vi "Q14070-Z120主界面.vi"() -> ()   [LabVIEW 2013]
uses:
  PCI8622_32.dll
  <vilib>/printing/EasyPrintingControls.llb/report_type.ctl
  <vilib>/Utility/NIReport.llb/NI_ReportGenerationCore.lvlib
  <vilib>/printing/EasyPrintingControls.llb/contents.ctl
  <vilib>/Utility/NIReport.llb/NI_report.lvclass
  <vilib>/printing/EasyPrinting.llb/Easy Print VI Panel or Documentation (path).vi
panel:
  out "电压值":dbl format="%#_4g"
  in  "压力零点标定":dbl=1.7 format="%#_4g"
  out "右压力换向(N)":dbl=5000.0 format="%#.2f"
  out "左压力换向(N)":dbl=5000.0 format="%#.2f"
  out "右压力换向":bool
  out "左压力换向":bool
  out "气缸启用":dbl
  in  "型号数量":i32=2
  in  "光幕报警使能 2":bool
  in  "光幕报警工步":dbl
  out "光幕报警提示":string
  out "顶升压力":dbl
  out "右伺服顶升位置":dbl format="%#.2f"
  out "左伺服顶升位置":dbl format="%#.2f"
  out "右顶升压力合格":bool
  out "左顶升压力合格":bool
  out "保压时间":dbl
  out "error out":errorcluster
  out "右伺服压入深度上限(mm)":dbl format="%#.2f"
  out "右伺服压入深度下限(mm)":dbl format="%#.2f"
  out "右伺服压入力上限(N)":dbl format="%#.2f"
  out "右伺服压入力下限(N)":dbl format="%#.2f"
  out "左伺服压入深度上限(mm)":dbl format="%#.2f"
  out "左伺服压入深度下限(mm)":dbl format="%#.2f"
  out "左伺服压入力上限(N)":dbl format="%#.2f"
  out "左伺服压入力下限(N)":dbl format="%#.2f"
  out "查询上序完成":bool
  out "上序合格":bool
  out "上序完成":bool
  out "本序完成":bool
  out "本序合格":bool
  in  "产品ID字符位数":dbl
  out "压力报警1":bool
  out "压力报警2":bool
  out "伺服慢进速度":dbl
  out "右伺服慢进位置":dbl format="%#.2f"
  out "左伺服慢进位置":dbl format="%#.2f"
  out "JSSJ":string
  out "FGCS":string
  out "KSSJ":string
  out "右压力参数组":dbl[](array[numeric])
  out "右位移参数组":dbl[](array[numeric])
  out "左压力参数组":dbl[](array[numeric])
  out "左位移参数组":dbl[](array[numeric])
  out "右伺服设定走位":dbl
  out "左伺服设定走位":dbl
  out "程序选择-2":bool
  out "程序选择-1":bool
  out "工步提示2":string
  out "工步提示1":string
  in  "报警工步号":u32 caption="工步号1"
  out "报警提示":string
  in  "自动工步号":u32 caption="工步号1"
  out "自动工步提示":string
  in  "产品ID":string="201209190001"
  out "员工ID":string
  out "员工姓名":string
  in  "电动缸全回零":bool
  in  "电动缸全复位":bool
  out "右伺服快进位置":dbl format="%#.2f"
  out "左伺服快进位置":dbl format="%#.2f"
  out "伺服快进速度":dbl
  out "参数保存错误":errorcluster
  out "传感器保存错误":errorcluster
  out "左实时压力(N)":dbl format="%#.3f"
  out "左实时位移(mm)":dbl=10000.0 format="%#.2f"
  out "右实时位移(mm)":dbl=10000.0 format="%#.2f"
  out "右实时压力(N)":dbl format="%#.3f"
  out "区域最小压力(N)":dbl format="%#.3f"
  out "监控点最大压力(N)":dbl format="%#.3f"
  out "监控点最小压力(N)":dbl format="%#.3f"
  out "区域最大压力(N)":dbl format="%#.3f"
  out "区域最小位移(mm)":dbl format="%#.1f"
  out "区域最大位移(mm)":dbl format="%#.1f"
  in  "左工步号2900":u32 caption="工步号1"
  in  "右工步号2700":u32 caption="工步号"
  in  "报警清除":bool
  in  "参数加载":bool
  in  "型号选择":u32(ring) items=["J706", "J709", "J728"]
  out "参数加载错误":errorcluster
  in  "停止":bool
  out "ADODB._Connection Out":refnum<k7>
  out "参数查询错误":errorcluster
  in  "联线按钮":bool
  out "通讯状态":bool
  in  "选项卡控件":T1(tab)
  out "右区域最大压力(N)":dbl
  out "右区域最小压力(N)":dbl
  out "左区域最大压力(N)":dbl
  out "左区域最小压力(N)":dbl
  out "右实测压入压力(N)":dbl format="%#.1f"
  out "左实测压入压力(N)":dbl format="%#.1f"
  out "左压力位移曲线":cluster{"Y":dbl[], "Y":dbl[]}[](graph)=[{"Y"=array[1892 elements], "Y"=array[1892 elements]}, {"Y"=[120.0, 145.0, 145.0, 120.0, 120.0], "Y"=[0.0, 0.0, 4000.0, 4000.0, 0.0]}] caption="XY图"
  out "右压力位移曲线":cluster{"Y":dbl[], "Y":dbl[]}[](graph)=[{"Y"=array[1892 elements], "Y"=array[1892 elements]}, {"Y"=[120.0, 145.0, 145.0, 120.0, 120.0], "Y"=[0.0, 0.0, 4000.0, 4000.0, 0.0]}] caption="XY图"
  out "左实测监控点压力(N)":dbl format="%#.3f"
  out "左实测压入位移(mm)":dbl format="%#.1f"
  out "右实测压入位移(mm)":dbl format="%#.1f"
  out "右实测监控点压力(N)":dbl format="%#.3f"
  out "监控点位移(mm)":dbl format="%#.2f"
  out "左压装合格":bool
  out "左压装不合格":bool
  out "右压装不合格":bool
  out "右压装合格":bool
  out "右电动缸零位":bool
  out "左电动缸下限":bool
  out "右气缸下降":bool
  out "右气缸上升":bool
  out "右气缸下位":bool
  out "右气缸上位":bool
  out "左气缸上升":bool
  out "左气缸下降":bool
  out "左气缸上位":bool
  out "左气缸下位":bool
  out "左电动缸零位":bool
  out "右电动缸上限":bool
  out "右电动缸下限":bool
  out "左电动缸上限":bool
  in  "顶升气缸上升-右":bool
  in  "顶升气缸下降-右":bool
  in  "顶升气缸上升-左":bool
  in  "顶升气缸下降-左":bool
  out "启动2按钮":bool
  out "启动1按钮":bool
  out "手动/自动":bool
  out "复位按钮":bool
  in  "电动缸下降-右":bool
  in  "电动缸上升-右":bool
  in  "电动缸下降-左":bool
  in  "电动缸上升-左":bool
  in  "电动缸回零-右":bool
  in  "电动缸回零-左":bool
  in  "电动缸复位-左":bool
  in  "电动缸复位-右":bool
  out "急停按钮":bool
  out "安全光幕":bool
  out "气压报警":bool
  in  "光幕报警使能":bool
  in  "右伺服设定走位":dbl caption="右伺服设定走位负值"
  in  "左伺服设定走位":dbl caption="左伺服设定走位负值"
  in  "电动缸绝对移动调试-右":bool
  in  "电动缸绝对移动调试-左":bool
  out "左伺服实时位置":dbl
  out "右伺服实时位置":dbl
  in  "电动缸复位-右 2":bool
  in  "电动缸复位-左 2":bool
  in  "电动缸回零-左 2":bool
  in  "电动缸回零-右 2":bool
  in  "电动缸下降-右 2":bool
  in  "电动缸上升-右 2":bool
  in  "电动缸下降-左 2":bool
  in  "电动缸上升-左 2":bool
  out "J709减震套批次号输入成功":bool
  out "J706右减震套批次号输入成功":bool
  out "J706左减震套批次号输入成功":bool
  in  "J709减震套批次号":string
  in  "J706右减震套批次号":string
  in  "J706左减震套批次号":string
  in  "传感器参数保存":bool
  in  "压力1零点偏移值":dbl format="%#.3f"
  in  "压力1比例偏移值":dbl format="%#.3f"
  in  "左位移比例偏移值":dbl format="%#.3f"
  in  "左位移零点偏移值":dbl format="%#.3f"
  in  "压力2零点偏移值":dbl format="%#.3f"
  in  "压力2比例偏移值":dbl format="%#.3f"
  in  "右位移比例偏移值":dbl format="%#.3f"
  in  "右位移零点偏移值":dbl format="%#.3f"
  in  "参数保存":bool
  in  "参数查询":bool
  in  "参数列表":string[][](table)
  # "压减震套"
  # "Copying (C) 2014 湖北唯思凌科装备制造有限公司 版权所有"
  # "此界面供伺服定位用，正常生产时 禁止操作！！！"
  # "批次号输入成功"
  # "传感器校验区"
  # "关于传感器校验：\n1、传感器校验需要由具备资质的单位或部门进行校验。\n2、具备权限的用户才能够修改传感器校验参数和试验参数。\n3、修改校验参数方法：先将比例偏移置为1，修改零点偏移，使零点值与校验的传感器一致；然后根据增幅调整比例偏移。"
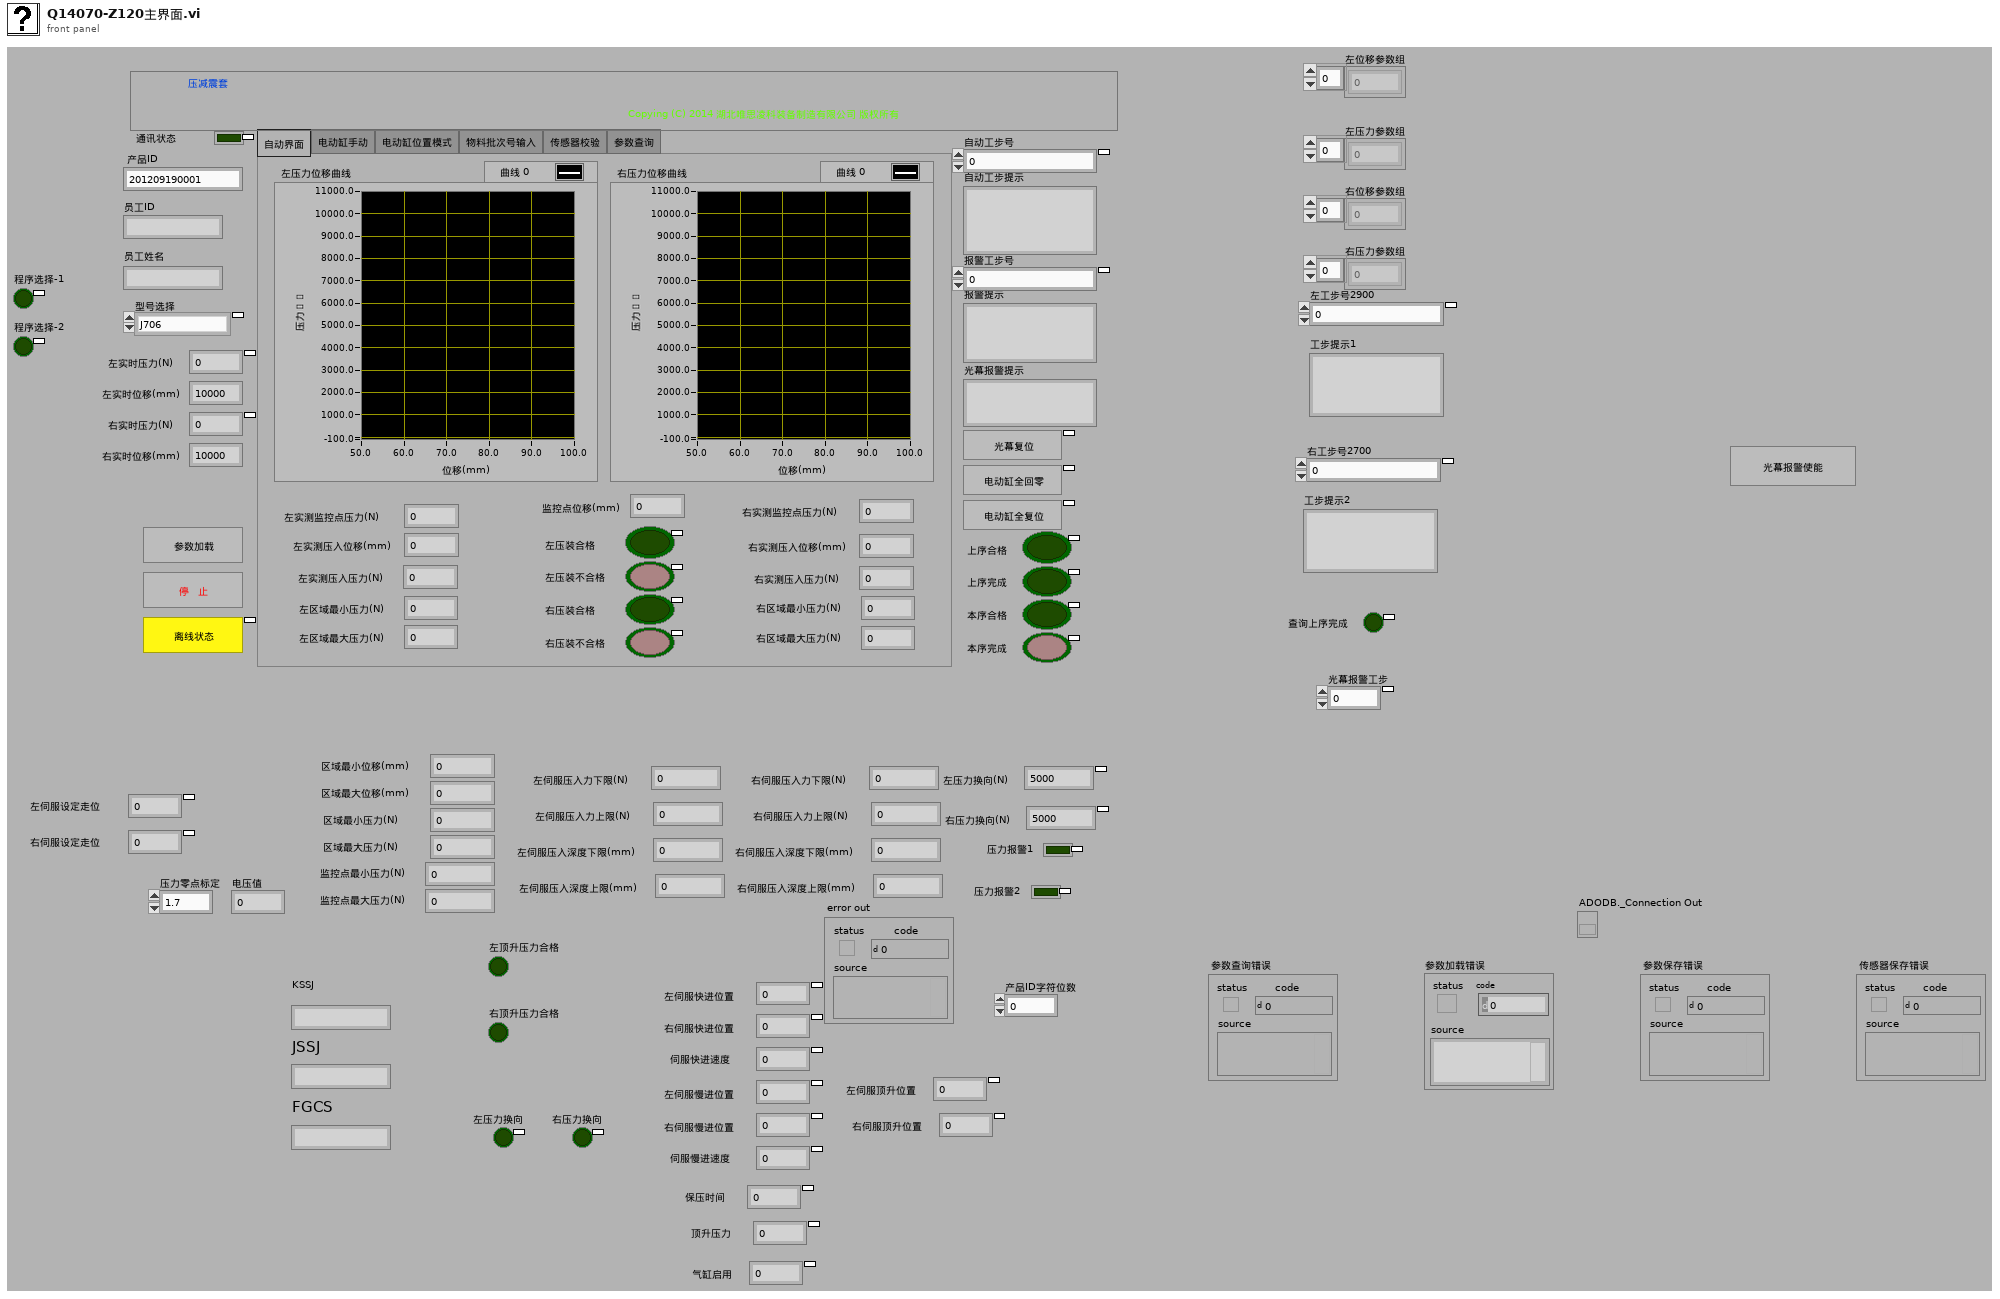
[diagram p1: front panel]
types:
  T1 = enum32{"自动界面", "电动缸手动", "电动缸位置模式", "物料批次号输入", "传感器校验", "参数查询"}
  T2 = typedef "NI_ReportGenerationCore.lvlib/report_type.ctl" = u16
  T3 = typedef "NI_ReportGenerationCore.lvlib/contents.ctl" = u16
  T4 = typedef "imagedata.ctl" = cluster{"image type":i32, "image depth":i32, "image":u8[], "mask":u8[], "colors":u32[], "Rectangle":cluster{"left":i16, "top":i16, "right":i16, "bottom":i16}}
  T5 = enum32{"invalid app kind", "Development System", "Run Time System", "Student Edition", "Embedded LabVIEW", "Evaluation", "Custom"}
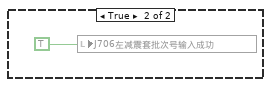
[diagram p3: hidden frame]
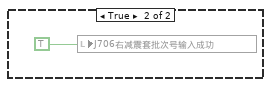
[diagram p4: hidden frame]
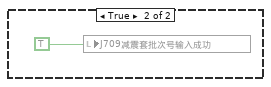
[diagram p5: hidden frame]
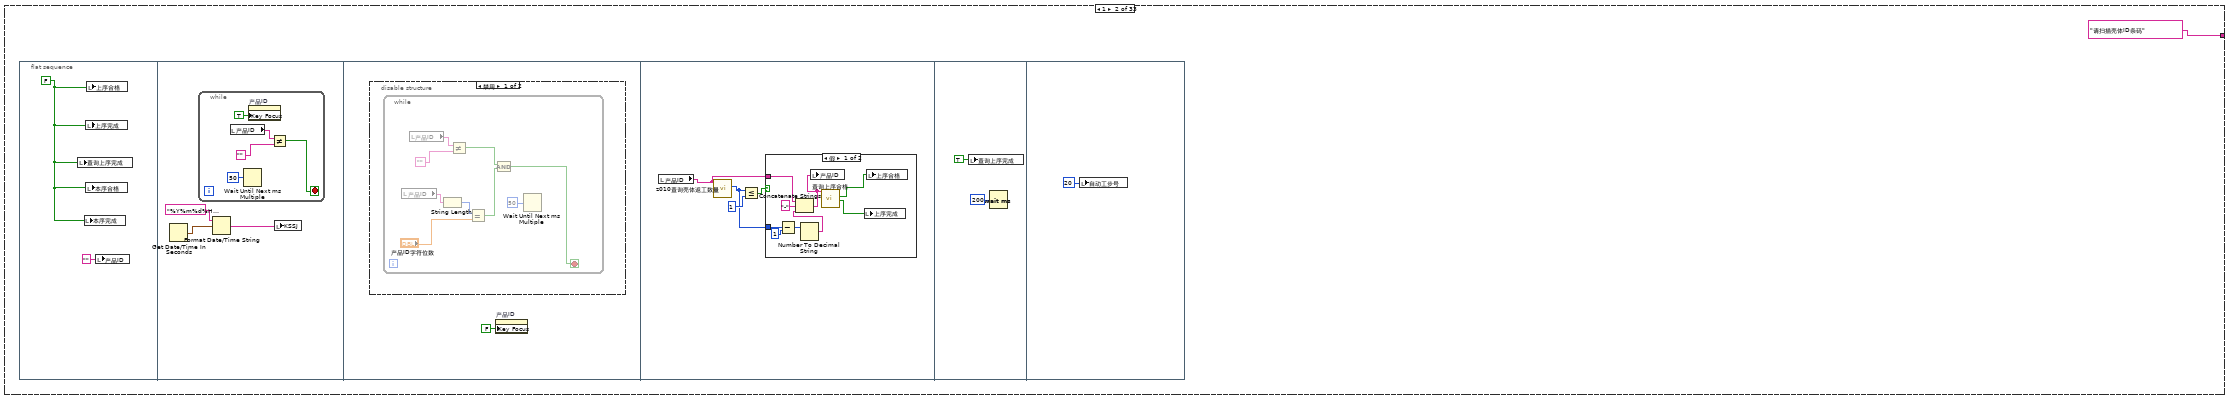
[diagram p8: hidden frame]
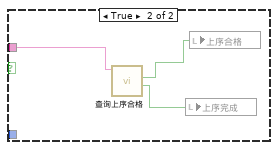
[diagram p10: hidden frame]
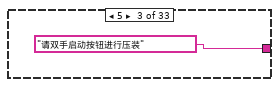
[diagram p11: hidden frame]
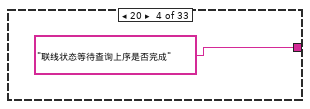
[diagram p12: hidden frame]
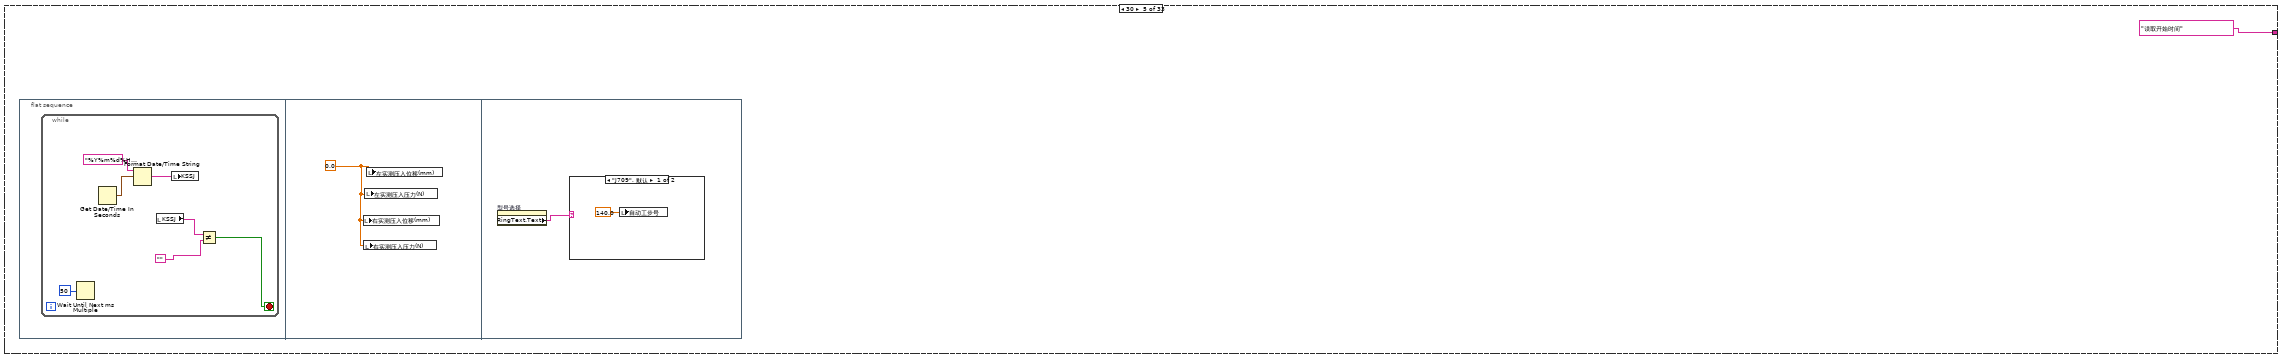
[diagram p13: hidden frame]
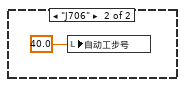
[diagram p14: hidden frame]
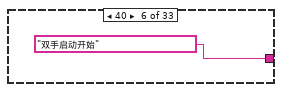
[diagram p15: hidden frame]
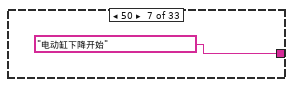
[diagram p16: hidden frame]
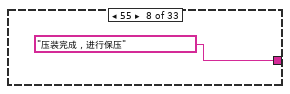
[diagram p17: hidden frame]
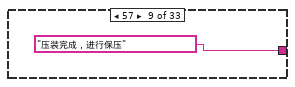
[diagram p18: hidden frame]
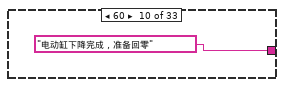
[diagram p19: hidden frame]
diagram:
  n1 = disable-structure shown="禁用" {
    frame Disabled {
      n2 = while {
        stop <- FALSE stop-if-true
        n3 = local read "右实时压力(N)"() -> (w10:dbl)
        n4 = local read "右工步号2700"() -> (w6:u32)
        n5 = local read "左实时压力(N)"() -> (w16:dbl)
        n6 = local read "左工步号2900"() -> (w18:u32)
        n7 = Greater Or Equal?(x=w16, y=1500.0) -> (x >= y?=w13:bool)
        n8 = Equal?(x=w18, y=u32 45) -> (x = y?=w14:bool)
        n9 = Greater Or Equal?(x=w10, y=1500.0) -> (x >= y?=w9:bool)
        n10 = Equal?(x=w6, y=u32 45) -> (x = y?=w5:bool)
        n11 = Compound Arithmetic op=AND(w5, w9) -> (→"右顶升压力合格":bool)
        n12 = Compound Arithmetic op=AND(w14, w13) -> (→"左顶升压力合格":bool)
      }
    }
    frame Enabled {
    }
  }
  n13 = while {
    stop <- w21 stop-if-true
    n14 = property on="型号选择" class="Ring (严格)"() -> ("RingText.Text"=w19:string)  [unwired: 2 in, 2 out]
    n15 = local read "停止"() -> (w21:bool)
    n16 = Wait Until Next ms Multiple(millisecond multiple=u32 50 ("毫秒倍数")) -> ()  [unwired: 1 out]
    n17 = case shown="\"J728\"" w19 {
      frame "J709", Default {
        n18 = local read "右工步号2700"() -> (w22:u32)
        n19 = case shown="20" w22 {
          frame 0, Default {
          }
          frame 20 {
            n20 = flat-sequence {
              tunnel: [w27] -> w23
              tunnel: [w34] -> w25
              tunnel: [w33] -> w24
              tunnel: w23 -> [w32]
              tunnel: w25 -> [w52]
              tunnel: w24 -> [w51]
              frame #0 {
                w26 = FALSE ("压装合格2")
                n21 = local write "右压装合格"(w26) -> ()
                n22 = local write "右压装不合格"(w26) -> ()
              }
              frame #1 {
                n23 = local read "区域最小位移(mm)"() -> (w31:dbl)
                n24 = local read "区域最大位移(mm)"() -> (w30:dbl)
                n25 = local read "区域最小压力(N)"() -> (w29:dbl)
                n26 = local read "区域最大压力(N)"() -> (w28:dbl)
                n27 = call "区域曲线.vi"("区域最大压力(N)"=w28, "区域最小压力(N)"=w29, "区域最大位移(mm)"=w30, "区域最小位移(mm)"=w31) -> ("区域曲线"=w27:cluster{dbl[], dbl[]})  [unwired: 7 in]
              }
              frame #2 {
                w35 = dbl[] []
                n28 = while {
                  shift-right: [w46] -> w34
                  shift-left: w35 -> [w47]
                  shift-right: [w44] -> w33
                  shift-left: w35 -> [w45]
                  tunnel: w32 -> [w37]
                  stop <- w41 stop-if-true
                  n29 = local read "左实时压力(N)"() -> (w39:dbl)
                  n30 = local read "左实时位移(mm)"() -> (w38:dbl)
                  n31 = local read "右工步号2700"() -> (w43:u32)
                  n32 = Build Array (concatenate)(w47, w38) -> (w46:dbl[])
                  n33 = Build Array (concatenate)(w45, w39) -> (w44:dbl[])
                  n34 = Equal?(x=w43, y=30.0) -> (x = y?=w41:bool)
                  n35 = Bundle(w46, w44) -> (w48:cluster{dbl[], dbl[]})  [unwired: 1 in]
                  n36 = Build Array(w48, w37) -> (w36:cluster{dbl[], dbl[]}[])
                  n37 = local write "右压力位移曲线"(w36) -> ()
                  n38 = Wait Until Next ms Multiple(millisecond multiple=u32 50 ("毫秒倍数")) -> ()  [unwired: 1 out]
                }
              }
              frame #3 {
                n39 = local read "监控点位移(mm)"() -> (w53:dbl)
                n40 = local write "右压力参数组"(w51) -> ()
                n41 = local write "右位移参数组"(w52) -> ()
                n42 = Array Max & Min "数组最大值与最小值"(array=w52) -> (max value=w50:dbl)  [unwired: 3 out]
                n43 = call "压力位移插值.vi"("压力数组"=w51, "监控点位移"=w53, "位移数组"=w52) -> ("监控点压力"=w49:dbl)  [unwired: 2 in]
                n44 = local write "右实测压入位移(mm)"(w50) -> ()
                n45 = local write "右实测监控点压力(N)"(w49) -> ()
              }
              frame #4 {
                n46 = local read "右实测压入位移(mm)"() -> (w55:dbl)
                n47 = local read "右位移参数组"() -> (w57:dbl[])
                n48 = local read "右压力参数组"() -> (w56:dbl[])
                n49 = call "压力位移插值.vi"("压力数组"=w56, "监控点位移"=w55, "位移数组"=w57) -> ("监控点压力"=w54:dbl)  [unwired: 2 in]
                n50 = local write "右实测压入压力(N)"(w54) -> ()
              }
              frame #5 {
                n51 = local read "右伺服压入力上限(N)"() -> (w63:dbl)
                n52 = local read "右伺服压入深度下限(mm)"() -> (w62:dbl)
                n53 = local read "右伺服压入力下限(N)"() -> (w65:dbl)
                n54 = local read "右实测压入压力(N)"() -> (w64:dbl)
                n55 = local read "右伺服压入深度上限(mm)"() -> (w60:dbl)
                n56 = local read "右实测压入位移(mm)"() -> (w61:dbl)
                n57 = Less Or Equal?(x=w65, y=w64) -> (x <= y?=w66:bool)
                n58 = Less Or Equal?(x=w64, y=w63) -> (x <= y?=w67:bool)
                n59 = Less Or Equal?(x=w62, y=w61) -> (x <= y?=w68:bool)
                n60 = Less Or Equal?(x=w61, y=w60) -> (x <= y?=w69:bool)
                n61 = Compound Arithmetic op=AND(w66, w67, w68, w69) -> (w59:bool)
                n62 = Not(x=w59) -> (.not. x?=w58:bool)
                n63 = local write "右压装不合格"(w58) -> ()
                n64 = local write "右压装合格"(w59) -> ()
              }
              frame #6 {
                n65 = local write "右工步号2700"(40.0 ("工步2序号")) -> ()
              }
            }
          }
        }
      }
      frame "J728" {
        n66 = local read "右工步号2700"() -> (w71:u32)
        n67 = case shown="20" w71 {
          frame 0, Default {
          }
          frame 20 {
            n68 = flat-sequence {
              tunnel: [w76] -> w72
              tunnel: [w83] -> w74
              tunnel: [w82] -> w73
              tunnel: w72 -> [w81]
              tunnel: w74 -> [w101]
              tunnel: w73 -> [w100]
              frame #0 {
                w75 = FALSE ("压装合格2")
                n69 = local write "右压装合格"(w75) -> ()
                n70 = local write "右压装不合格"(w75) -> ()
              }
              frame #1 {
                n71 = local read "区域最小位移(mm)"() -> (w80:dbl)
                n72 = local read "区域最大位移(mm)"() -> (w79:dbl)
                n73 = local read "区域最小压力(N)"() -> (w78:dbl)
                n74 = local read "区域最大压力(N)"() -> (w77:dbl)
                n75 = call "区域曲线.vi"("区域最大压力(N)"=w77, "区域最小压力(N)"=w78, "区域最大位移(mm)"=w79, "区域最小位移(mm)"=w80) -> ("区域曲线"=w76:cluster{dbl[], dbl[]})  [unwired: 7 in]
              }
              frame #2 {
                w84 = dbl[] []
                n76 = while {
                  shift-right: [w95] -> w83
                  shift-left: w84 -> [w96]
                  shift-right: [w93] -> w82
                  shift-left: w84 -> [w94]
                  tunnel: w81 -> [w90]
                  stop <- w85 stop-if-true
                  n77 = local read "右实时压力(N)"() -> (w91:dbl)
                  n78 = local read "右实时位移(mm)"() -> (w88:dbl)
                  n79 = local read "右压力换向(N)"() -> (w87:dbl)
                  n80 = local read "右实时压力(N)"() -> (w86:dbl)
                  n81 = Build Array (concatenate)(w96, w88) -> (w95:dbl[])
                  n82 = Build Array (concatenate)(w94, w91) -> (w93:dbl[])
                  n83 = Greater Or Equal?(x=w86, y=w87) -> (x >= y?=w85:bool)
                  n84 = Bundle(w95, w93) -> (w97:cluster{dbl[], dbl[]})  [unwired: 1 in]
                  n85 = local write "右压力换向"(w85) -> ()
                  n86 = Build Array(w97, w90) -> (w89:cluster{dbl[], dbl[]}[])
                  n87 = local write "右压力位移曲线"(w89) -> ()
                  n88 = Wait Until Next ms Multiple(millisecond multiple=u32 50 ("毫秒倍数")) -> ()  [unwired: 1 out]
                }
              }
              frame #3 {
                n89 = local read "区域最小位移(mm)"() -> (w105:dbl)
                n90 = local read "区域最大位移(mm)"() -> (w104:dbl)
                n91 = local read "监控点位移(mm)"() -> (w108:dbl)
                n92 = local read "区域最小压力(N)"() -> (w103:dbl)
                n93 = local read "区域最大压力(N)"() -> (w102:dbl)
                n94 = local write "右压力参数组"(w100) -> ()
                n95 = local write "右位移参数组"(w101) -> ()
                n96 = Array Max & Min "数组最大值与最小值"(array=w101) -> (max value=w107:dbl)  [unwired: 3 out]
                n97 = call "压力位移插值.vi"("压力数组"=w100, "监控点位移"=w108, "位移数组"=w101) -> ("监控点压力"=w106:dbl)  [unwired: 2 in]
                n98 = call "区域判断.vi"("压力数组"=w100, "位移数组"=w101, "区域最大压力"=w102, "区域最小压力"=w103, "区域最大位移"=w104, "区域最小位移"=w105) -> ("数值 2"=→"右区域最小压力(N)":dbl, "数值"=→"右区域最大压力(N)":dbl)  [unwired: 1 in, 1 out]
                n99 = local write "右实测压入位移(mm)"(w107) -> ()
                n100 = local write "右实测监控点压力(N)"(w106) -> ()
              }
              frame #4 {
                n101 = local read "右实测压入位移(mm)"() -> (w110:dbl)
                n102 = local read "右位移参数组"() -> (w112:dbl[])
                n103 = local read "右压力参数组"() -> (w111:dbl[])
                n104 = call "压力位移插值.vi"("压力数组"=w111, "监控点位移"=w110, "位移数组"=w112) -> ("监控点压力"=w109:dbl)  [unwired: 2 in]
                n105 = local write "右实测压入压力(N)"(w109) -> ()
              }
              frame #5 {
                n106 = local read "右伺服压入力上限(N)"() -> (w118:dbl)
                n107 = local read "右伺服压入深度下限(mm)"() -> (w117:dbl)
                n108 = local read "右伺服压入力下限(N)"() -> (w120:dbl)
                n109 = local read "右实测压入压力(N)"() -> (w119:dbl)
                n110 = local read "右伺服压入深度上限(mm)"() -> (w115:dbl)
                n111 = local read "右实测压入位移(mm)"() -> (w116:dbl)
                n112 = Less Or Equal?(x=w120, y=w119) -> (x <= y?=w121:bool)
                n113 = Less Or Equal?(x=w119, y=w118) -> (x <= y?=w122:bool)
                n114 = Less Or Equal?(x=w117, y=w116) -> (x <= y?=w123:bool)
                n115 = Less Or Equal?(x=w116, y=w115) -> (x <= y?=w124:bool)
                n116 = Compound Arithmetic op=AND(w121, w122, w123, w124) -> (w114:bool)
                n117 = Not(x=w114) -> (.not. x?=w113:bool)
                n118 = local write "右压装不合格"(w113) -> ()
                n119 = local write "右压装合格"(w114) -> ()
              }
              frame #6 {
                n120 = local write "右工步号2700"(40.0 ("工步2序号")) -> ()
              }
            }
          }
        }
      }
      frame "J706" {
        n121 = local read "右工步号2700"() -> (w126:u32)
        n122 = case shown="20" w126 {
          frame 0, Default {
          }
          frame 20 {
            n123 = flat-sequence {
              tunnel: [w131] -> w127
              tunnel: [w138] -> w129
              tunnel: [w137] -> w128
              tunnel: w127 -> [w136]
              tunnel: w129 -> [w156]
              tunnel: w128 -> [w155]
              frame #0 {
                w130 = FALSE ("压装合格2")
                n124 = local write "右压装合格"(w130) -> ()
                n125 = local write "右压装不合格"(w130) -> ()
              }
              frame #1 {
                n126 = local read "区域最小位移(mm)"() -> (w135:dbl)
                n127 = local read "区域最大位移(mm)"() -> (w134:dbl)
                n128 = local read "区域最小压力(N)"() -> (w133:dbl)
                n129 = local read "区域最大压力(N)"() -> (w132:dbl)
                n130 = call "区域曲线.vi"("区域最大压力(N)"=w132, "区域最小压力(N)"=w133, "区域最大位移(mm)"=w134, "区域最小位移(mm)"=w135) -> ("区域曲线"=w131:cluster{dbl[], dbl[]})  [unwired: 7 in]
              }
              frame #2 {
                w139 = dbl[] []
                n131 = while {
                  shift-right: [w150] -> w138
                  shift-left: w139 -> [w151]
                  shift-right: [w148] -> w137
                  shift-left: w139 -> [w149]
                  tunnel: w136 -> [w145]
                  stop <- w142 stop-if-true
                  n132 = local read "右工步号2700"() -> (w141:u32)
                  n133 = local read "右实时压力(N)"() -> (w146:dbl)
                  n134 = local read "右实时位移(mm)"() -> (w143:dbl)
                  n135 = Build Array (concatenate)(w151, w143) -> (w150:dbl[])
                  n136 = Build Array (concatenate)(w149, w146) -> (w148:dbl[])
                  n137 = Equal?(x=w141, y=30) -> (x = y?=w142:bool)
                  n138 = Bundle(w150, w148) -> (w152:cluster{dbl[], dbl[]})  [unwired: 1 in]
                  n139 = Build Array(w152, w145) -> (w144:cluster{dbl[], dbl[]}[])
                  n140 = local write "右压力位移曲线"(w144) -> ()
                  n141 = Wait Until Next ms Multiple(millisecond multiple=u32 50 ("毫秒倍数")) -> ()  [unwired: 1 out]
                }
              }
              frame #3 {
                n142 = local read "区域最小位移(mm)"() -> (w160:dbl)
                n143 = local read "区域最大位移(mm)"() -> (w159:dbl)
                n144 = local read "监控点位移(mm)"() -> (w163:dbl)
                n145 = local read "区域最小压力(N)"() -> (w158:dbl)
                n146 = local read "区域最大压力(N)"() -> (w157:dbl)
                n147 = local write "右压力参数组"(w155) -> ()
                n148 = local write "右位移参数组"(w156) -> ()
                n149 = Array Max & Min "数组最大值与最小值"(array=w156) -> (max value=w162:dbl)  [unwired: 3 out]
                n150 = call "压力位移插值.vi"("压力数组"=w155, "监控点位移"=w163, "位移数组"=w156) -> ("监控点压力"=w161:dbl)  [unwired: 2 in]
                n151 = call "区域判断.vi"("压力数组"=w155, "位移数组"=w156, "区域最大压力"=w157, "区域最小压力"=w158, "区域最大位移"=w159, "区域最小位移"=w160) -> ("数值 2"=w153:dbl, "数值"=w154:dbl)  [unwired: 1 in, 1 out]
                n152 = local write "右实测压入位移(mm)"(w162) -> ()
                n153 = local write "右实测监控点压力(N)"(w161) -> ()
                n154 = local write "右区域最大压力(N)"(w154) -> ()
                n155 = local write "右区域最小压力(N)"(w153) -> ()
              }
              frame #4 {
                n156 = local read "右实测压入位移(mm)"() -> (w165:dbl)
                n157 = local read "右位移参数组"() -> (w167:dbl[])
                n158 = local read "右压力参数组"() -> (w166:dbl[])
                n159 = call "压力位移插值.vi"("压力数组"=w166, "监控点位移"=w165, "位移数组"=w167) -> ("监控点压力"=w164:dbl)  [unwired: 2 in]
                n160 = local write "右实测压入压力(N)"(w164) -> ()
              }
              frame #5 {
                n161 = local read "右伺服压入力上限(N)"() -> (w173:dbl)
                n162 = local read "右伺服压入深度下限(mm)"() -> (w172:dbl)
                n163 = local read "右伺服压入力下限(N)"() -> (w175:dbl)
                n164 = local read "右实测压入压力(N)"() -> (w174:dbl)
                n165 = local read "右伺服压入深度上限(mm)"() -> (w170:dbl)
                n166 = local read "右实测压入位移(mm)"() -> (w171:dbl)
                n167 = Less Or Equal?(x=w175, y=w174) -> (x <= y?=w176:bool)
                n168 = Less Or Equal?(x=w174, y=w173) -> (x <= y?=w177:bool)
                n169 = Less Or Equal?(x=w172, y=w171) -> (x <= y?=w178:bool)
                n170 = Less Or Equal?(x=w171, y=w170) -> (x <= y?=w179:bool)
                n171 = Compound Arithmetic op=AND(w176, w177, w178, w179) -> (w169:bool)
                n172 = Not(x=w169) -> (.not. x?=w168:bool)
                n173 = local write "右压装不合格"(w168) -> ()
                n174 = local write "右压装合格"(w169) -> ()
              }
              frame #6 {
                n175 = local write "右工步号2700"(40.0 ("工步2序号")) -> ()
              }
            }
          }
        }
      }
    }
  }
  n176 = while {
    stop <- w183 stop-if-true
    n177 = property on="型号选择" class="Ring (严格)"() -> ("RingText.Text"=w181:string)  [unwired: 2 in, 2 out]
    n178 = Wait Until Next ms Multiple(millisecond multiple=u32 50 ("毫秒倍数")) -> ()  [unwired: 1 out]
    n179 = local read "停止"() -> (w183:bool)
    n180 = case shown="\"J706\"" w181 {
      frame "J709", Default {
        n181 = local read "左工步号2900"() -> (w184:u32)
        n182 = case shown="20" w184 {
          frame 0, Default {
          }
          frame 20 {
            n183 = flat-sequence {
              tunnel: [w193] -> w187
              tunnel: [w196] -> w186
              tunnel: [w195] -> w185
              tunnel: w187 -> [w194]
              tunnel: w186 -> [w214]
              tunnel: w185 -> [w213]
              frame #0 {
                w188 = FALSE ("压装合格1")
                n184 = local write "左压装不合格"(w188) -> ()
                n185 = local write "左压装合格"(w188) -> ()
              }
              frame #1 {
                n186 = local read "区域最小位移(mm)"() -> (w192:dbl)
                n187 = local read "区域最大位移(mm)"() -> (w191:dbl)
                n188 = local read "区域最小压力(N)"() -> (w190:dbl)
                n189 = local read "区域最大压力(N)"() -> (w189:dbl)
                n190 = call "区域曲线.vi"("区域最大压力(N)"=w189, "区域最小压力(N)"=w190, "区域最大位移(mm)"=w191, "区域最小位移(mm)"=w192) -> ("区域曲线"=w193:cluster{dbl[], dbl[]})  [unwired: 7 in]
              }
              frame #2 {
                w197 = dbl[] []
                n191 = while {
                  shift-right: [w208] -> w196
                  shift-left: w197 -> [w209]
                  shift-right: [w206] -> w195
                  shift-left: w197 -> [w207]
                  tunnel: w194 -> [w199]
                  stop <- w201 stop-if-true
                  n192 = local read "左实时位移(mm)"() -> (w205:dbl)
                  n193 = local read "左工步号2900"() -> (w203:u32)
                  n194 = local read "左实时压力(N)"() -> (w204:dbl)
                  n195 = Build Array (concatenate)(w209, w205) -> (w208:dbl[])
                  n196 = Build Array (concatenate)(w207, w204) -> (w206:dbl[])
                  n197 = Equal?(x=w203, y=30.0) -> (x = y?=w201:bool)
                  n198 = Bundle(w208, w206) -> (w210:cluster{dbl[], dbl[]})  [unwired: 1 in]
                  n199 = Build Array(w210, w199) -> (w198:cluster{dbl[], dbl[]}[])
                  n200 = local write "左压力位移曲线"(w198) -> ()
                  n201 = Wait Until Next ms Multiple(millisecond multiple=u32 50 ("毫秒倍数")) -> ()  [unwired: 1 out]
                }
              }
              frame #3 {
                n202 = local read "监控点位移(mm)"() -> (w216:dbl)
                n203 = local write "左位移参数组"(w214) -> ()
                n204 = local write "左压力参数组"(w213) -> ()
                n205 = Array Max & Min "数组最大值与最小值"(array=w214) -> (max value=w212:dbl)  [unwired: 3 out]
                n206 = call "压力位移插值.vi"("压力数组"=w213, "监控点位移"=w216, "位移数组"=w214) -> ("监控点压力"=w211:dbl)  [unwired: 2 in]
                n207 = local write "左实测监控点压力(N)"(w211) -> ()
                n208 = local write "左实测压入位移(mm)"(w212) -> ()
                n209 = Wait (ms)(milliseconds to wait=u32 200 ("等待时间（毫秒）")) -> ()  [unwired: 1 out]
              }
              frame #4 {
                n210 = local read "左实测压入位移(mm)"() -> (w218:dbl)
                n211 = local read "左位移参数组"() -> (w220:dbl[])
                n212 = local read "左压力参数组"() -> (w219:dbl[])
                n213 = call "压力位移插值.vi"("压力数组"=w219, "监控点位移"=w218, "位移数组"=w220) -> ("监控点压力"=w217:dbl)  [unwired: 2 in]
                n214 = local write "左实测压入压力(N)"(w217) -> ()
              }
              frame #5 {
                n215 = local read "左实测压入压力(N)"() -> (w224:dbl)
                n216 = local read "左伺服压入力下限(N)"() -> (w232:dbl)
                n217 = local read "左伺服压入力上限(N)"() -> (w231:dbl)
                n218 = local read "左伺服压入深度下限(mm)"() -> (w225:dbl)
                n219 = local read "左实测压入位移(mm)"() -> (w221:dbl)
                n220 = local read "左伺服压入深度上限(mm)"() -> (w230:dbl)
                n221 = Less Or Equal?(x=w232, y=w224) -> (x <= y?=w229:bool)
                n222 = Less Or Equal?(x=w224, y=w231) -> (x <= y?=w228:bool)
                n223 = Less Or Equal?(x=w225, y=w221) -> (x <= y?=w227:bool)
                n224 = Less Or Equal?(x=w221, y=w230) -> (x <= y?=w226:bool)
                n225 = Compound Arithmetic op=AND(w229, w228, w227, w226) -> (w223:bool)
                n226 = Not(x=w223) -> (.not. x?=w222:bool)
                n227 = local write "左压装合格"(w223) -> ()
                n228 = local write "左压装不合格"(w222) -> ()
              }
              frame #6 {
                n229 = local write "左工步号2900"(40.0 ("工步2序号")) -> ()
              }
            }
          }
        }
      }
      frame "J728" {
        n230 = local read "左工步号2900"() -> (w234:u32)
        n231 = case shown="20" w234 {
          frame 0, Default {
          }
          frame 20 {
            n232 = flat-sequence {
              tunnel: [w243] -> w235
              tunnel: [w246] -> w237
              tunnel: [w245] -> w236
              tunnel: w235 -> [w244]
              tunnel: w237 -> [w264]
              tunnel: w236 -> [w263]
              frame #0 {
                w238 = FALSE ("压装合格1")
                n233 = local write "左压装不合格"(w238) -> ()
                n234 = local write "左压装合格"(w238) -> ()
              }
              frame #1 {
                n235 = local read "区域最小位移(mm)"() -> (w242:dbl)
                n236 = local read "区域最大位移(mm)"() -> (w241:dbl)
                n237 = local read "区域最小压力(N)"() -> (w240:dbl)
                n238 = local read "区域最大压力(N)"() -> (w239:dbl)
                n239 = call "区域曲线.vi"("区域最大压力(N)"=w239, "区域最小压力(N)"=w240, "区域最大位移(mm)"=w241, "区域最小位移(mm)"=w242) -> ("区域曲线"=w243:cluster{dbl[], dbl[]})  [unwired: 7 in]
              }
              frame #2 {
                w247 = dbl[] []
                n240 = while {
                  shift-right: [w258] -> w246
                  shift-left: w247 -> [w259]
                  shift-right: [w256] -> w245
                  shift-left: w247 -> [w257]
                  tunnel: w244 -> [w252]
                  stop <- w248 stop-if-true
                  n241 = local read "左实时位移(mm)"() -> (w255:dbl)
                  n242 = local read "左实时压力(N)"() -> (w249:dbl)
                  n243 = local read "左实时压力(N)"() -> (w254:dbl)
                  n244 = local read "左压力换向(N)"() -> (w250:dbl)
                  n245 = Build Array (concatenate)(w259, w255) -> (w258:dbl[])
                  n246 = Build Array (concatenate)(w257, w254) -> (w256:dbl[])
                  n247 = Greater Or Equal?(x=w249, y=w250) -> (x >= y?=w248:bool)
                  n248 = local write "左压力换向"(w248) -> ()
                  n249 = Bundle(w258, w256) -> (w260:cluster{dbl[], dbl[]})  [unwired: 1 in]
                  n250 = Build Array(w260, w252) -> (w251:cluster{dbl[], dbl[]}[])
                  n251 = local write "左压力位移曲线"(w251) -> ()
                  n252 = Wait Until Next ms Multiple(millisecond multiple=u32 50 ("毫秒倍数")) -> ()  [unwired: 1 out]
                }
              }
              frame #3 {
                n253 = local read "监控点位移(mm)"() -> (w272:dbl)
                n254 = local read "区域最小压力(N)"() -> (w266:dbl)
                n255 = local read "区域最大压力(N)"() -> (w265:dbl)
                n256 = local read "区域最小位移(mm)"() -> (w268:dbl)
                n257 = local read "区域最大位移(mm)"() -> (w267:dbl)
                n258 = local write "左位移参数组"(w264) -> ()
                n259 = local write "左压力参数组"(w263) -> ()
                n260 = Array Max & Min "数组最大值与最小值"(array=w264) -> (max value=w270:dbl)  [unwired: 3 out]
                n261 = call "压力位移插值.vi"("压力数组"=w263, "监控点位移"=w272, "位移数组"=w264) -> ("监控点压力"=w269:dbl)  [unwired: 2 in]
                n262 = call "区域判断.vi"("压力数组"=w263, "位移数组"=w264, "区域最大压力"=w265, "区域最小压力"=w266, "区域最大位移"=w267, "区域最小位移"=w268) -> ("数值 2"=→"左区域最小压力(N)":dbl, "数值"=→"左区域最大压力(N)":dbl)  [unwired: 1 in, 1 out]
                n263 = local write "左实测监控点压力(N)"(w269) -> ()
                n264 = local write "左实测压入位移(mm)"(w270) -> ()
                n265 = Wait (ms)(milliseconds to wait=u32 200 ("等待时间（毫秒）")) -> ()  [unwired: 1 out]
              }
              frame #4 {
                n266 = local read "左实测压入位移(mm)"() -> (w274:dbl)
                n267 = local read "左位移参数组"() -> (w276:dbl[])
                n268 = local read "左压力参数组"() -> (w275:dbl[])
                n269 = call "压力位移插值.vi"("压力数组"=w275, "监控点位移"=w274, "位移数组"=w276) -> ("监控点压力"=w273:dbl)  [unwired: 2 in]
                n270 = local write "左实测压入压力(N)"(w273) -> ()
              }
              frame #5 {
                n271 = local read "左实测压入压力(N)"() -> (w280:dbl)
                n272 = local read "左伺服压入力下限(N)"() -> (w288:dbl)
                n273 = local read "左伺服压入力上限(N)"() -> (w287:dbl)
                n274 = local read "左伺服压入深度下限(mm)"() -> (w281:dbl)
                n275 = local read "左实测压入位移(mm)"() -> (w277:dbl)
                n276 = local read "左伺服压入深度上限(mm)"() -> (w286:dbl)
                n277 = Less Or Equal?(x=w288, y=w280) -> (x <= y?=w285:bool)
                n278 = Less Or Equal?(x=w280, y=w287) -> (x <= y?=w284:bool)
                n279 = Less Or Equal?(x=w281, y=w277) -> (x <= y?=w283:bool)
                n280 = Less Or Equal?(x=w277, y=w286) -> (x <= y?=w282:bool)
                n281 = Compound Arithmetic op=AND(w285, w284, w283, w282) -> (w279:bool)
                n282 = Not(x=w279) -> (.not. x?=w278:bool)
                n283 = local write "左压装合格"(w279) -> ()
                n284 = local write "左压装不合格"(w278) -> ()
              }
              frame #6 {
                n285 = local write "左工步号2900"(40.0 ("工步2序号")) -> ()
              }
            }
          }
        }
      }
      frame "J706" {
        n286 = local read "左工步号2900"() -> (w290:u32)
        n287 = case shown="20" w290 {
          frame 0, Default {
          }
          frame 20 {
            n288 = flat-sequence {
              tunnel: [w299] -> w291
              tunnel: [w302] -> w293
              tunnel: [w301] -> w292
              tunnel: w291 -> [w300]
              tunnel: w293 -> [w320]
              tunnel: w292 -> [w319]
              frame #0 {
                w294 = FALSE ("压装合格1")
                n289 = local write "左压装不合格"(w294) -> ()
                n290 = local write "左压装合格"(w294) -> ()
              }
              frame #1 {
                n291 = local read "区域最小位移(mm)"() -> (w298:dbl)
                n292 = local read "区域最大位移(mm)"() -> (w297:dbl)
                n293 = local read "区域最小压力(N)"() -> (w296:dbl)
                n294 = local read "区域最大压力(N)"() -> (w295:dbl)
                n295 = call "区域曲线.vi"("区域最大压力(N)"=w295, "区域最小压力(N)"=w296, "区域最大位移(mm)"=w297, "区域最小位移(mm)"=w298) -> ("区域曲线"=w299:cluster{dbl[], dbl[]})  [unwired: 7 in]
              }
              frame #2 {
                w303 = dbl[] []
                n296 = while {
                  shift-right: [w314] -> w302
                  shift-left: w303 -> [w315]
                  shift-right: [w312] -> w301
                  shift-left: w303 -> [w313]
                  tunnel: w300 -> [w308]
                  stop <- w306 stop-if-true
                  n297 = local read "左实时位移(mm)"() -> (w311:dbl)
                  n298 = local read "左工步号2900"() -> (w304:u32)
                  n299 = local read "左实时压力(N)"() -> (w310:dbl)
                  n300 = Build Array (concatenate)(w315, w311) -> (w314:dbl[])
                  n301 = Build Array (concatenate)(w313, w310) -> (w312:dbl[])
                  n302 = Equal?(x=w304, y=30.0) -> (x = y?=w306:bool)
                  n303 = Bundle(w314, w312) -> (w316:cluster{dbl[], dbl[]})  [unwired: 1 in]
                  n304 = Build Array(w316, w308) -> (w307:cluster{dbl[], dbl[]}[])
                  n305 = local write "左压力位移曲线"(w307) -> ()
                  n306 = Wait Until Next ms Multiple(millisecond multiple=u32 50 ("毫秒倍数")) -> ()  [unwired: 1 out]
                }
              }
              frame #3 {
                n307 = local read "监控点位移(mm)"() -> (w328:dbl)
                n308 = local read "区域最小压力(N)"() -> (w322:dbl)
                n309 = local read "区域最大压力(N)"() -> (w321:dbl)
                n310 = local read "区域最小位移(mm)"() -> (w324:dbl)
                n311 = local read "区域最大位移(mm)"() -> (w323:dbl)
                n312 = local write "左位移参数组"(w320) -> ()
                n313 = local write "左压力参数组"(w319) -> ()
                n314 = Array Max & Min "数组最大值与最小值"(array=w320) -> (max value=w326:dbl)  [unwired: 3 out]
                n315 = call "压力位移插值.vi"("压力数组"=w319, "监控点位移"=w328, "位移数组"=w320) -> ("监控点压力"=w325:dbl)  [unwired: 2 in]
                n316 = call "区域判断.vi"("压力数组"=w319, "位移数组"=w320, "区域最大压力"=w321, "区域最小压力"=w322, "区域最大位移"=w323, "区域最小位移"=w324) -> ("数值 2"=w317:dbl, "数值"=w318:dbl)  [unwired: 1 in, 1 out]
                n317 = local write "左实测监控点压力(N)"(w325) -> ()
                n318 = local write "左实测压入位移(mm)"(w326) -> ()
                n319 = Wait (ms)(milliseconds to wait=u32 200 ("等待时间（毫秒）")) -> ()  [unwired: 1 out]
                n320 = local write "左区域最大压力(N)"(w318) -> ()
                n321 = local write "左区域最小压力(N)"(w317) -> ()
              }
              frame #4 {
                n322 = local read "左实测压入位移(mm)"() -> (w330:dbl)
                n323 = local read "左位移参数组"() -> (w332:dbl[])
                n324 = local read "左压力参数组"() -> (w331:dbl[])
                n325 = call "压力位移插值.vi"("压力数组"=w331, "监控点位移"=w330, "位移数组"=w332) -> ("监控点压力"=w329:dbl)  [unwired: 2 in]
                n326 = local write "左实测压入压力(N)"(w329) -> ()
              }
              frame #5 {
                n327 = local read "左实测压入压力(N)"() -> (w336:dbl)
                n328 = local read "左伺服压入力下限(N)"() -> (w344:dbl)
                n329 = local read "左伺服压入力上限(N)"() -> (w343:dbl)
                n330 = local read "左伺服压入深度下限(mm)"() -> (w337:dbl)
                n331 = local read "左实测压入位移(mm)"() -> (w333:dbl)
                n332 = local read "左伺服压入深度上限(mm)"() -> (w342:dbl)
                n333 = Less Or Equal?(x=w344, y=w336) -> (x <= y?=w341:bool)
                n334 = Less Or Equal?(x=w336, y=w343) -> (x <= y?=w340:bool)
                n335 = Less Or Equal?(x=w337, y=w333) -> (x <= y?=w339:bool)
                n336 = Less Or Equal?(x=w333, y=w342) -> (x <= y?=w338:bool)
                n337 = Compound Arithmetic op=AND(w341, w340, w339, w338) -> (w335:bool)
                n338 = Not(x=w335) -> (.not. x?=w334:bool)
                n339 = local write "左压装合格"(w335) -> ()
                n340 = local write "左压装不合格"(w334) -> ()
              }
              frame #6 {
                n341 = local write "左工步号2900"(40.0 ("工步2序号")) -> ()
              }
            }
          }
        }
      }
    }
  }
  n342 = while {
    stop <- w348 stop-if-true
    n343 = Wait Until Next ms Multiple(millisecond multiple=u32 50 ("毫秒倍数")) -> ()  [unwired: 1 out]
    n344 = local read "自动工步号"() -> (w349:u32)
    n345 = local read "停止"() -> (w348:bool)
    n346 = case shown="0, 默认" w349 {
      tunnel: ["请扫描物料批次号" "请扫描壳体ID条码" "请双手启动按钮进行压装" "联线状态等待查询上序是否完成" "读取开始时间" "双手启动开始" "电动缸下降开始" "压装完成，进行保压" "压装完成，进行保压" "电动缸下降完成，准备回零" _ "等待左右伺服缸回零中" "" "" "" "" "" _ "" "" "" "" "" "" "" _ "" "" "" "绘制保存曲线、参数" "上传数据至服务器" "循环完成，归零" "联线状态查询上序不合格，请返修"] -> w346
      frame 0, Default {
        w350 = FALSE ("右压力换向")
        n347 = disable-structure shown="禁用" {
          frame Disabled {
            n348 = flat-sequence {
              frame #0 {
                n349 = while {
                  stop <- w354 stop-if-true
                  n350 = local read "J706左减震套批次号"() -> (w353:string)
                  n351 = local read "自动工步号"() -> (w352:u32)
                  n352 = Not Equal?(x=w353, y="") -> (x != y?=w356:bool)
                  n353 = Not Equal?(x=w352, y=0.0) -> (x != y?=w355:bool)
                  n354 = Compound Arithmetic op=OR(w356, w355) -> (w354:bool)
                  n355 = Wait Until Next ms Multiple(millisecond multiple=u32 50 ("毫秒倍数")) -> ()  [unwired: 1 out]
                }
              }
              frame #1 {
                n356 = local read "J706左减震套批次号"() -> (w362:string)
                n357 = property on="型号选择" class="Ring (严格)"() -> ("RingText.Text"=w360:string)  [unwired: 2 in, 2 out]
                n358 = call "比较批次号关键字.vi"("批次号"=w362, "外购件名称"="", "产品型号"=w360) -> ("关键字正确"=w361:bool)  [unwired: 6 in, 1 out]
                n359 = case shown="假" w361 {
                  frame False {
                    n360 = local write "J706左减震套批次号输入成功"(FALSE ("防尘罩批次号输入成功")) -> ()
                    n361 = call "显示对话框信息"("Enable"=TRUE) -> ()  [unwired: 9 in, 2 out]
                    n362 = local write "J706左减震套批次号"("") -> ()
                  }
                  frame True {
                    n363 = local write "J706左减震套批次号输入成功"(TRUE ("防尘罩批次号输入成功")) -> ()
                  }
                }
              }
              frame #2 {
                n364 = while {
                  stop <- w370 stop-if-true
                  n365 = local read "J706右减震套批次号"() -> (w369:string)
                  n366 = local read "自动工步号"() -> (w368:u32)
                  n367 = Not Equal?(x=w369, y="") -> (x != y?=w372:bool)
                  n368 = Not Equal?(x=w368, y=0.0) -> (x != y?=w371:bool)
                  n369 = Compound Arithmetic op=OR(w372, w371) -> (w370:bool)
                  n370 = Wait Until Next ms Multiple(millisecond multiple=u32 50 ("毫秒倍数")) -> ()  [unwired: 1 out]
                }
              }
              frame #3 {
                n371 = local read "J706右减震套批次号"() -> (w377:string)
                n372 = property on="型号选择" class="Ring (严格)"() -> ("RingText.Text"=w379:string)  [unwired: 2 in, 2 out]
                n373 = call "比较批次号关键字.vi"("批次号"=w377, "外购件名称"="", "产品型号"=w379) -> ("关键字正确"=w378:bool)  [unwired: 6 in, 1 out]
                n374 = case shown="假" w378 {
                  frame False {
                    n375 = local write "J706右减震套批次号输入成功"(FALSE ("防尘罩批次号输入成功")) -> ()
                    n376 = call "显示对话框信息4"("Enable"=TRUE) -> ()  [unwired: 9 in, 2 out]
                    n377 = local write "J706右减震套批次号"("") -> ()
                  }
                  frame True {
                    n378 = local write "J706右减震套批次号输入成功"(TRUE ("防尘罩批次号输入成功")) -> ()
                  }
                }
              }
              frame #4 {
                n379 = while {
                  stop <- w388 stop-if-true
                  n380 = local read "J709减震套批次号"() -> (w387:string)
                  n381 = local read "自动工步号"() -> (w385:u32)
                  n382 = Not Equal?(x=w385, y=0.0) -> (x != y?=w384:bool)
                  n383 = Not Equal?(x=w387, y="") -> (x != y?=w389:bool)
                  n384 = Wait Until Next ms Multiple(millisecond multiple=u32 50 ("毫秒倍数")) -> ()  [unwired: 1 out]
                  n385 = Compound Arithmetic op=OR(w389, w384) -> (w388:bool)
                }
              }
              frame #5 {
                n386 = local read "J709减震套批次号"() -> (w393:string)
                n387 = property on="型号选择" class="Ring (严格)"() -> ("RingText.Text"=w395:string)  [unwired: 2 in, 2 out]
                n388 = call "比较批次号关键字.vi"("批次号"=w393, "外购件名称"="", "产品型号"=w395) -> ("关键字正确"=w394:bool)  [unwired: 6 in, 1 out]
                n389 = case shown="假" w394 {
                  frame False {
                    n390 = local write "J709减震套批次号输入成功"(FALSE ("防尘罩批次号输入成功")) -> ()
                    n391 = call "显示对话框信息3"("Enable"=TRUE) -> ()  [unwired: 9 in, 2 out]
                    n392 = local write "J709减震套批次号"("") -> ()
                  }
                  frame True {
                    n393 = local write "J709减震套批次号输入成功"(TRUE ("防尘罩批次号输入成功")) -> ()
                  }
                }
              }
              frame #6 {
                n394 = local read "J706左减震套批次号输入成功"() -> (w403:bool)
                n395 = local read "J706右减震套批次号输入成功"() -> (w401:bool)
                n396 = local read "J709减震套批次号输入成功"() -> (w400:bool)
                n397 = Compound Arithmetic op=AND(w403, w401, w400) -> (w402:bool)
                n398 = case shown="真" w402 {
                  frame False {
                  }
                  frame True {
                    n399 = local write "自动工步号"(1.0 ("批次号扫描工步")) -> ()
                  }
                }
              }
            }
          }
          frame Enabled {
          }
        }
        n400 = local write "右压力换向"(w350) -> ()
        n401 = local write "左压力换向"(w350) -> ()
      }
      frame 1 {
        n402 = flat-sequence {
          frame #0 {
            w407 = FALSE ("上序合格")
            n403 = local write "查询上序完成"(w407) -> ()
            n404 = local write "本序完成"(w407) -> ()
            n405 = local write "上序完成"(w407) -> ()
            n406 = local write "本序合格"(w407) -> ()
            n407 = local write "上序合格"(w407) -> ()
            n408 = local write "产品ID"("" ("产品ID")) -> ()
          }
          frame #1 {
            n409 = Get Date/Time In Seconds() -> (seconds since 1Jan1904=w410:timestamp)
            n410 = while {
              stop <- w411 stop-if-true
              n411 = local read "产品ID"() -> (w412:string)
              n412 = Wait Until Next ms Multiple(millisecond multiple=u32 50 ("毫秒倍数")) -> ()  [unwired: 1 out]
              n413 = property on="产品ID" class="Str"("Key Focus"=TRUE ("键选中")) -> ()  [unwired: 2 in, 2 out]
              n414 = Not Equal?(x=w412, y="") -> (x != y?=w411:bool)
            }
            n415 = Format Date/Time String(time format string (%c)="%Y%m%d%H%M" ("时间格式字符串(%c)"), seconds (now)=w410) -> (date/time string=w408:string)  [unwired: 1 in]
            n416 = local write "KSSJ"(w408) -> ()
          }
          frame #2 {
            n417 = disable-structure shown="禁用" {
              frame Disabled {
                n418 = while {
                  stop <- w419 stop-if-true
                  n419 = local read "产品ID"() -> (w423:string)
                  n420 = local read "产品ID"() -> (w425:string)
                  n421 = String Length(string=w423) -> (length=w422:i32)
                  n422 = Not Equal?(x=w425, y="") -> (x != y?=w420:bool)
                  n423 = Equal?(x=w422, y="产品ID字符位数") -> (x = y?=w421:bool)
                  n424 = Compound Arithmetic op=AND(w420, w421) -> (w419:bool)
                  n425 = Wait Until Next ms Multiple(millisecond multiple=u32 50 ("毫秒倍数")) -> ()  [unwired: 1 out]
                }
              }
              frame Enabled {
              }
            }
            n426 = property on="产品ID" class="Str"("Key Focus"=FALSE ("键选中")) -> ()  [unwired: 2 in, 2 out]
          }
          frame #3 {
            n427 = local read "产品ID"() -> (w427:string)
            n428 = call "z010查询壳体返工数量.vi"("转向器总成ID"=w427) -> ("Rows Fetched"=w426:i32)  [unwired: 8 in, 2 out]
            n429 = Less Or Equal?(x=w426, y=1) -> (x <= y?=w429:bool)
            n430 = case shown="假" w429 {
              tunnel: w427 -> [w432 w439]
              tunnel: w426 -> [w435 _]
              frame False {
                n431 = Subtract(x=w435, y=1) -> (x-y=w433:i32)
                n432 = Number To Decimal String(number=w433) -> (decimal integer string=w436:string)  [unwired: 1 in]
                n433 = Concatenate Strings(w432, "-" ("字符串"), w436) -> (w430:string)
                n434 = local write "产品ID"(w430) -> ()
                n435 = call "查询上序合格.vi"("产品ID"=w430) -> ("本序已做"=w438:bool, "上序合格"=w437:bool)  [unwired: 8 in, 1 out]
                n436 = local write "上序完成"(w438) -> ()
                n437 = local write "上序合格"(w437) -> ()
              }
              frame True {
                n438 = call "查询上序合格.vi"("产品ID"=w439) -> ("本序已做"=w441:bool, "上序合格"=w440:bool)  [unwired: 8 in, 1 out]
                n439 = local write "上序完成"(w441) -> ()
                n440 = local write "上序合格"(w440) -> ()
              }
            }
          }
          frame #4 {
            n441 = local write "查询上序完成"(TRUE ("查询上序完成")) -> ()
            n442 = Wait (ms)(milliseconds to wait=u32 200 ("等待时间（毫秒）")) -> ()  [unwired: 1 out]
          }
          frame #5 {
            n443 = local write "自动工步号"(u32 20 ("自动工步号")) -> ()
          }
        }
      }
      frame 5 {
      }
      frame 20 {
      }
      frame 30 {
        n444 = flat-sequence {
          frame #0 {
            n445 = while {
              stop <- w448 stop-if-true
              n446 = Wait Until Next ms Multiple(millisecond multiple=u32 50 ("毫秒倍数")) -> ()  [unwired: 1 out]
              n447 = Get Date/Time In Seconds() -> (seconds since 1Jan1904=w453:timestamp)
              n448 = Format Date/Time String(time format string (%c)="%Y%m%d%H%M" ("时间格式字符串(%c)"), seconds (now)=w453) -> (date/time string=w452:string)  [unwired: 1 in]
              n449 = local read "KSSJ"() -> (w450:string)
              n450 = local write "KSSJ"(w452) -> ()
              n451 = Not Equal?(x=w450, y="") -> (x != y?=w448:bool)
            }
          }
          frame #1 {
            w455 = 0.0 ("左实测压入位移(mm)")
            n452 = local write "右实测压入位移(mm)"(w455) -> ()
            n453 = local write "右实测压入压力(N)"(w455) -> ()
            n454 = local write "左实测压入压力(N)"(w455) -> ()
            n455 = local write "左实测压入位移(mm)"(w455) -> ()
          }
          frame #2 {
            n456 = property on="型号选择" class="Ring (严格)"() -> ("RingText.Text"=w456:string)  [unwired: 2 in, 2 out]
            n457 = case shown="\"J709\", 默认" w456 {
              frame "J709", Default {
                n458 = local write "自动工步号"(140.0 ("内球节工步号")) -> ()
              }
              frame "J706" {
                n459 = local write "自动工步号"(40.0 ("内球节工步号")) -> ()
              }
            }
          }
        }
      }
      frame 40 {
      }
      frame 50 {
      }
      frame 55 {
      }
      frame 57 {
      }
      frame 60 {
      }
      frame 65 {
      }
      frame 70 {
      }
      frame 140 {
      }
      frame 150 {
      }
      frame 155 {
      }
      frame 157 {
      }
      frame 160 {
      }
      frame 165 {
      }
      frame 170 {
      }
      frame 180 {
      }
      frame 240 {
      }
      frame 250 {
      }
      frame 255 {
      }
      frame 257 {
      }
      frame 260 {
      }
      frame 265 {
      }
      frame 270 {
      }
      frame 280 {
      }
      frame 290 {
      }
      frame 800 {
        n460 = flat-sequence {
          tunnel: [w510] -> w499
          tunnel: [w508] -> w498
          tunnel: [w502] -> w483
          tunnel: [w500] -> w480
          tunnel: w499 -> [w517]
          tunnel: w498 -> [w516]
          tunnel: [w517] -> w497
          tunnel: [w516] -> w496
          tunnel: ["F:\\报表存储\\" ("字符串")] -> w495
          tunnel: w483 -> [w514]
          tunnel: [w514] -> w482
          tunnel: [w513] -> w481
          tunnel: w480 -> [w513]
          tunnel: w497 -> [w522]
          tunnel: w496 -> [w518]
          tunnel: w495 -> [w523]
          tunnel: [w532] -> w494
          tunnel: [w530] -> w493
          tunnel: [w528] -> w492
          tunnel: [w524] -> w491
          tunnel: w482 -> [w521]
          tunnel: w481 -> [w520]
          tunnel: w494 -> [w538]
          tunnel: [w539] -> w490
          tunnel: w493 -> [w539]
          tunnel: w492 -> [w537]
          tunnel: [w536] -> w489
          tunnel: w491 -> [w535]
          tunnel: [w534] -> w488
          tunnel: [w553] -> w487
          tunnel: w490 -> [w553]
          tunnel: w489 -> [w552]
          tunnel: [w552] -> w486
          tunnel: [w551] -> w485
          tunnel: w488 -> [w551]
          tunnel: w487 -> [w560]
          tunnel: w486 -> [w559]
          tunnel: w485 -> [w556]
          frame #0 {
            n461 = local read "产品ID"() -> (w509:string)
            n462 = Format Date/Time String(time format string (%c)="%Y%m%d" ("时间格式字符串(%c)")) -> (date/time string=w501:string)  [unwired: 2 in]
            n463 = String Subset(string=w501, offset (0)=4 ("偏移量(0)"), length (rest)=2 ("长度（剩余）")) -> (substring=w502:string)
            n464 = String Subset(string=w501, offset (0)=6 ("偏移量(0)"), length (rest)=2 ("长度（剩余）")) -> (substring=w500:string)
            n465 = call <vilib>:"Trim Whitespace.vi"("string"=w509) -> ("trimmed string"=w508:string)  [unwired: 1 in]
            n466 = String Subset(string=w501, offset (0)=0 ("偏移量(0)"), length (rest)=4 ("长度（剩余）")) -> (substring=w510:string)
          }
          frame #1 {
          }
          frame #2 {
            w519 = "\\" ("字符串")
            n467 = Concatenate Strings(w523, w522, w519, w521, w519, w520, w519) -> (w525:string)
            n468 = Concatenate Strings(w523, w522, w519, w521, w519, w520, w519) -> (w533:string)
            n469 = String To Path(string=w533) -> (path=w532:path)
            n470 = Concatenate Strings(w525, w518, ".JPG" ("字符串")) -> (w531:string)
            n471 = Concatenate Strings(w525, w518, "右.txt" ("字符串")) -> (w524:string)
            n472 = Concatenate Strings(w525, w518, "左.txt" ("字符串")) -> (w528:string)
            n473 = String To Path(string=w531) -> (path=w530:path)
          }
          frame #3 {
            n474 = call <vilib>:"Check if File or Folder Exists.vi"("path"=w538) -> ("file or folder exists?"=w540:bool)  [unwired: 8 in, 2 out]
            n475 = String To Path(string=w537) -> (path=w536:path)
            n476 = String To Path(string=w535) -> (path=w534:path)
            n477 = case shown="真" w540 {
              tunnel: w538 -> [w541 w542]
              frame False {
                n478 = Create Folder(path (use dialog)=w541) -> ()  [unwired: 2 in, 3 out]
              }
              frame True {
                n479 = flat-sequence {
                  tunnel: w542 -> [w546]
                  tunnel: [w544] -> w543
                  tunnel: w543 -> [w549]
                  frame #0 {
                    n480 = Delete(path (use dialog)=w546, entire hierarchy (F)=TRUE ("整个层次结构(F)")) -> (deleted path=w544:path)  [unwired: 3 in, 2 out]
                  }
                  frame #1 {
                    n481 = call <vilib>:"Check if File or Folder Exists.vi"("path"=w549) -> ("file or folder exists?"=w548:bool, "dup path"=w547:path)  [unwired: 8 in, 1 out]
                    n482 = case shown="假" w548 {
                      tunnel: w547 -> [w550 _]
                      frame False {
                        n483 = Create Folder(path (use dialog)=w550) -> ()  [unwired: 2 in, 3 out]
                      }
                      frame True {
                      }
                    }
                  }
                }
              }
            }
          }
          frame #4 {
            n484 = Wait Until Next ms Multiple(millisecond multiple=u32 1000 ("毫秒倍数")) -> ()  [unwired: 1 out]
          }
          frame #5 {
            n485 = flat-sequence {
              tunnel: w559 -> [w563]
              tunnel: w560 -> [w564]
              tunnel: [w564] -> w558
              tunnel: [w563] -> w557
              tunnel: w556 -> [w562]
              tunnel: [w562] -> w555
              tunnel: w558 -> [w565]
              tunnel: w557 -> [w568]
              tunnel: w555 -> [w571]
              frame #0 {
                n486 = local write "选项卡控件"(T1."自动界面" ("选项卡控件")) -> ()
              }
              frame #1 {
                n487 = local read "左位移参数组"() -> (w572:dbl[])
                n488 = local read "左压力参数组"() -> (w573:dbl[])
                n489 = local read "右位移参数组"() -> (w569:dbl[])
                n490 = local read "右压力参数组"() -> (w570:dbl[])
                n491 = disable-structure shown="禁用" {
                  disable-tunnel: w565 -> [w574 _]
                  frame Disabled {
                    w577 = T2 2 items=["快速打印", "标准报表", "HTML", "双字节", "Excel"] ("report type (Quick Print)")
                    w576 = T3 1 items=["完整前面板", "前面板可见部分", "图标、说明、前面板和程序框图", "说明信息: 使用前面板", "说明信息: 作为子VI使用", "说明信息: 完整", "说明信息: 自定义"] ("contents (complete front panel)")
                    n492 = Current VI's Path() -> (path=w575:path)
                    n493 = call-poly <vilib>:"Easy Print VI Panel or Documentation.vi"("report type (Quick Print)"=w577, "contents (complete front panel)"=w576, "VI path"=w575) -> ("error out"=w579:errorcluster, "report out"=w578:refnum<class "NI_report.lvclass">)  [unwired: 1 in, 6 out]
                    n494 = call-dynamic "Save Report to File.vi"("report in"=w578, "report file path"=w574, "error in (no error)"=w579) -> ()  [unwired: 2 in, 11 out]
                  }
                  frame Enabled {
                  }
                }
                n495 = call "导出曲线数组.vi"("压力参数"=w573, "位移参数"=w572, "file path (dialog if empty)"=w568) -> ()  [unwired: 17 in]
                n496 = call "导出曲线数组.vi"("压力参数"=w570, "位移参数"=w569, "file path (dialog if empty)"=w571) -> ()  [unwired: 17 in]
                n497 = control-ref of="本VI"() -> (w567:refnum<vi>)
                n498 = invoke class="VI" method="FP.Get Image"(reference=w567) -> ("image data"=w566:T4)  [unwired: 5 in, 5 out]
                n499 = call <vilib>:"Write JPEG File.vi"("image data"=w566, "path to JPEG file"=w565) -> ()  [unwired: 8 in, 2 out]
              }
            }
          }
          frame #6 {
            n500 = local write "自动工步号"(810.0 ("工步号")) -> ()
          }
        }
      }
      frame 810 {
        n501 = flat-sequence {
          tunnel: [w609] -> w582
          tunnel: w582 -> [w617]
          frame #0 {
            n502 = while {
              stop <- w585 stop-if-true
              n503 = Get Date/Time In Seconds() -> (seconds since 1Jan1904=w590:timestamp)
              n504 = local read "JSSJ"() -> (w587:string)
              n505 = Format Date/Time String(time format string (%c)="%Y%m%d%H%M" ("时间格式字符串(%c)"), seconds (now)=w590) -> (date/time string=w588:string)  [unwired: 1 in]
              n506 = Wait Until Next ms Multiple(millisecond multiple=u32 50 ("毫秒倍数")) -> ()  [unwired: 1 out]
              n507 = Not Equal?(x=w587, y="") -> (x != y?=w585:bool)
              n508 = local write "JSSJ"(w588) -> ()
            }
            n509 = Wait (ms)(milliseconds to wait=u32 2000 ("等待时间（毫秒）")) -> ()  [unwired: 1 out]
          }
          frame #1 {
            w607 = i16 4 ("精度(6)")
            n510 = local read "右实测压入位移(mm)"() -> (w597:dbl)
            n511 = local read "右实测压入压力(N)"() -> (w596:dbl)
            n512 = local read "左实测压入压力(N)"() -> (w598:dbl)
            n513 = local read "左实测压入位移(mm)"() -> (w599:dbl)
            n514 = local read "右压装合格"() -> (w591:bool)
            n515 = local read "左压装合格"() -> (w592:bool)
            n516 = local read "J706左减震套批次号"() -> (w602:string)
            n517 = local read "J709减震套批次号"() -> (w600:string)
            n518 = local read "J706右减震套批次号"() -> (w601:string)
            n519 = local read "员工ID"() -> (w613:string)
            n520 = local read "产品ID"() -> (w614:string)
            n521 = local read "KSSJ"() -> (w612:string)
            n522 = local read "JSSJ"() -> (w608:string)
            n523 = local read "FGCS"() -> (w611:string)
            n524 = And(x=w592, y=w591) -> (x .and. y?=w593:bool)
            n525 = Boolean To (0,1)(Boolean=w593) -> (0, 1=w616:i16)
            n526 = Number To Decimal String(number=w616, width (-)=i16 1 ("宽度(-)")) -> (decimal integer string=w594:string)
            n527 = Number To Fractional String(number=w599, precision (6)=w607) -> (F-format string=w606:string)  [unwired: 2 in]
            n528 = Number To Fractional String(number=w598, precision (6)=w607) -> (F-format string=w605:string)  [unwired: 2 in]
            n529 = Number To Fractional String(number=w597, precision (6)=w607) -> (F-format string=w604:string)  [unwired: 2 in]
            n530 = Number To Fractional String(number=w596, precision (6)=w607) -> (F-format string=w603:string)  [unwired: 2 in]
            n531 = Build Array(w614, w613, "1", w594, w612, w608, w611, "Q14070-Z120", w606, w605, w604, w603, w602, w601, w600) -> (w609:string[])
          }
          frame #2 {
            n532 = Wait (ms)(milliseconds to wait=u32 500 ("等待时间（毫秒）")) -> ()  [unwired: 1 out]
            n533 = call "数据库更新.vi"("设备号"="11", "数据"=w617) -> ()  [unwired: 13 in, 1 out]
          }
          frame #3 {
            n534 = local write "自动工步号"(820.0 ("工步号")) -> ()
          }
        }
      }
      frame 820 {
      }
      frame 900 {
      }
    }
    "自动工步提示" <- w346
  }
  n535 = while {
    stop <- w623 stop-if-true
    n536 = stacked-sequence {
      frame #0 {
        n537 = First Call?() -> (First Call?: T/F=w625:bool)
        n538 = case shown="真" w625 {
          frame False {
          }
          frame True {
            n539 = call "员工管理测试程序.vi"() -> ("员工姓名"=w631:string, "员工ID"=w630:string)  [unwired: 10 in]
            n540 = local write "员工ID"(w630) -> ()
            n541 = local write "员工姓名"(w631) -> ()
          }
        }
        n542 = Negate(x="右伺服设定走位") -> (-x=→"右伺服设定走位":dbl)
        n543 = Negate(x="左伺服设定走位") -> (-x=→"左伺服设定走位":dbl)
      }
      frame #1 {
        n544 = case shown="0, 默认" "报警工步号" {
          tunnel: ["工作正常" "气压报警，请检查气压" "压装过程触碰光幕，请复位后双手启动重新压装" "左压装不合格" "右压装不合格" "左压装压力过大报警" "右压装压力过大报警" "左伺服报警，请复位伺服电机" "右伺服报警，请复位伺服电机" "左伺服达到下极限，请复位后，手动点动上升离开下极限" "左伺服达到上极限，请复位后，手动点动下降离开上极限" "右伺服达到下极限，请复位后，手动点动上升离开下极限" "右伺服达到上极限，请复位后，手动点动下降离开上极限" "联线状态查询上序不合格，请返修"] -> w639
          frame 0, Default {
          }
          frame 1 {
          }
          frame 2 {
          }
          frame 6 {
          }
          frame 7 {
          }
          frame 8 {
          }
          frame 9 {
          }
          frame 11 {
          }
          frame 12 {
          }
          frame 21 {
          }
          frame 22 {
          }
          frame 23 {
          }
          frame 24 {
          }
          frame 41 {
          }
        }
        "报警提示" <- w639
        n545 = case shown="10" "左工步号2900" {
          tunnel: ["准备压装" "左伺服压装启动" "左伺服等待回零完成" "左伺服等待回零完成，等待右伺服回零完成" "左伺服压装中" "左伺服压装结束" "左伺服曲线采集完成" "左伺服回零开始" "左伺服回零中" "左伺服回零完成" "左伺服压装工作结束"] -> w638
          frame 0, Default {
          }
          frame 10 {
          }
          frame 15 {
          }
          frame 16 {
          }
          frame 20 {
          }
          frame 30 {
          }
          frame 40 {
          }
          frame 50 {
          }
          frame 60 {
          }
          frame 70 {
          }
          frame 80 {
          }
        }
        "工步提示1" <- w638
        n546 = case shown="80" "右工步号2700" {
          tunnel: ["准备压装" "右伺服压装启动" "右伺服等待回零完成" "右伺服等待回零完成，等待左伺服回零完成" "右伺服压装中" "右伺服压装结束" "右伺服曲线采集完成" "右伺服回零开始" "右伺服回零中" "右伺服回零完成" "右伺服压装工作结束"] -> w637
          frame 0, Default {
          }
          frame 10 {
          }
          frame 15 {
          }
          frame 16 {
          }
          frame 20 {
          }
          frame 30 {
          }
          frame 40 {
          }
          frame 50 {
          }
          frame 60 {
          }
          frame 70 {
          }
          frame 80 {
          }
        }
        "工步提示2" <- w637
        n547 = case shown="5" "光幕报警工步" {
          tunnel: ["工作正常" "压装过程触碰光幕，请再次启动"] -> w632
          frame 0, Default {
          }
          frame 5 {
          }
        }
        "光幕报警提示" <- w632
        n548 = property on="型号选择" class="Ring (严格)"() -> ("RingText.Text"=w634:string)  [unwired: 2 in, 2 out]
        n549 = case shown="\"J706\", 默认" w634 {
          frame "J706", Default {
            n550 = local write "程序选择-1"(TRUE ("程序选择-1")) -> ()
            n551 = local write "程序选择-2"(FALSE ("程序选择-2")) -> ()
          }
          frame "J709" {
            n552 = local write "程序选择-1"(FALSE ("程序选择-1")) -> ()
            n553 = local write "程序选择-2"(TRUE ("程序选择-2")) -> ()
          }
        }
      }
    }
    n554 = Wait (ms)(milliseconds to wait=u32 50 ("毫秒倍数")) -> ()  [unwired: 1 out]
    n555 = local read "停止"() -> (w623:bool)
  }
  n556 = while {
    stop <- w683 stop-if-true
    n557 = event shown="[1] \"参数查询\": 值改变" {
      selector: _ -> [_ _ _ _ _]
      dyn-events: _ -> [_ _ _ _ _]
      timeout: 500 -> [_ _ _ _ _]
      tunnel: [_ _ _ _ w807] -> w683
      event Timeout {
        n558 = event-data() -> ()  [unwired: 1 in, 3 out]
      }
      event "参数查询": Value Change {
        n559 = event-data() -> ()  [unwired: 1 in, 6 out]
        n560 = flat-sequence {
          tunnel: [w694] -> w686
          tunnel: [w691] -> w685
          tunnel: w686 -> [w698]
          tunnel: w685 -> [w697]
          frame #0 {
            n561 = call "字符串转换为数组.vi"("查询内容"=",产品型号,区域最小位移(mm),区域最大位移(mm),区域最小压力(N),区域最大压力(N),位移监控点(mm),左伺服压入力下限(N),左伺服压入力上限(N),左伺服压入深度下限(mm),左伺服压入深度上限(mm),右伺服压入力下限(N),右伺服压入力上限(N),右伺服压入深度下限(mm),右伺服压入深度上限(mm),左伺服快进位置(mm),右伺服快进位置(mm),伺服快进速度(mm/s),左伺服慢进位置(mm),右伺服慢进位置(mm),左伺服顶升位置(mm),右伺服顶升位置(mm),伺服慢进速度(mm/s),保压时间(ms),顶升压力(N),气缸启用,左压力换向(N),右压力换向(N)") -> ("列首"=w687:string[])  [unwired: 10 in]
            n562 = property on="参数列表" class="Tbl (严格)"("Row Headers[]"=w687) -> ()  [unwired: 2 in, 2 out]
          }
          frame #1 {
            w690 = 0 ("禁用的索引 (列)")
            n563 = local read "ADODB._Connection Out"() -> (w695:refnum<k7>)
            n564 = call "SQL Execute.vi"("Command Text"="select * from 测试参数表 ", "ADODB._Connection In"=w695) -> ("error out"=w694:errorcluster, "Data"=w696:string[][])  [unwired: 6 in, 2 out]
            n565 = Transpose 2D Array "二维数组转置"(2D array=w696) -> (transposed array=w691:string[][])
            n566 = Index Array(array=w691, index (col)=w690) -> (element=w692:string[])  [unwired: 1 in]
            n567 = Index Array(array=w691, index (col)=w690) -> (element=w689:string[])  [unwired: 1 in]
            n568 = property on="参数列表" class="Tbl (严格)"("Column Headers[]"=w692) -> ()  [unwired: 2 in, 2 out]
            n569 = Array Size(array=w689) -> ()  [unwired: 1 out]
          }
          frame #2 {
            n570 = local write "参数列表"(w697) -> ()
            "参数查询错误" <- w698
          }
        }
      }
      event "参数保存": Value Change {
        n571 = event-data() -> ()  [unwired: 1 in, 6 out]
        n572 = while {
          i -> [w700]
          stop <- w711 stop-if-true
          n573 = local read "型号数量"() -> (w699:i32)
          n574 = local read "参数列表"() -> (w702:string[][])
          n575 = Greater Or Equal?(x=w700, y=w699) -> (x >= y?=w711:bool)
          n576 = Wait Until Next ms Multiple(millisecond multiple=u32 100 ("毫秒倍数")) -> ()  [unwired: 1 out]
          n577 = Index Array "索引数组"(array=w702, index (col)=w700) -> (element=w703:string[])  [unwired: 1 in]
          n578 = stacked-sequence {
            seq-local: [w714 _] -> [_ w768]
            tunnel: w703 -> [w745 w773]
            tunnel: [_ w767] -> w701
            frame #0 {
              n579 = Index Array(array=w745, index #2=1 ("索引"), index #3=2 ("索引"), index #4=3 ("索引"), index #5=4 ("索引"), index #6=5 ("索引"), index #7=6 ("索引"), index #8=7 ("索引"), index #9=8 ("索引"), index #10=9 ("索引"), index #11=10 ("索引"), index #12=11 ("索引"), index #13=12 ("索引"), index #14=13 ("索引"), index #15=14 ("索引"), index #16=15 ("索引"), index #17=16 ("索引"), index #18=17 ("索引"), index #19=18 ("索引"), index #20=19 ("索引"), index #21=20 ("索引"), index #22=21 ("索引"), index #23=22 ("索引"), index #24=23 ("索引")) -> (element #2=w737:string, element #3=w736:string, element #4=w735:string, element #5=w734:string, element #6=w733:string, element #7=w732:string, element #8=w731:string, element #9=w730:string, element #10=w729:string, element #11=w728:string, element #12=w727:string, element #13=w726:string, element #14=w725:string, element #15=w724:string, element #16=w723:string, element #17=w722:string, element #18=w721:string, element #19=w720:string, element #20=w719:string, element #21=w718:string, element #22=w717:string, element #23=w716:string, element #24=w715:string)  [unwired: 2 in, 2 out]
              n580 = call "创建文本3"("区域最小位移"=w737, "区域最a大位移"=w736, "区域最小压力"=w735, "区域最大压力"=w734, "位移监控点"=w733, "左伺服压入力下限"=w732, "左伺服压入力上限"=w731, "左伺服压入深度下限"=w730, "左伺服压入深度上限"=w729, "右伺服压入力下限"=w728, "右伺服压入力上限"=w727, "右伺服压入深度下限"=w726, "右伺服压入深度上限"=w725, "左伺服快进位置"=w724, "右伺服快进位置"=w723, "伺服快进速度"=w722, "左伺服慢进位置"=w721, "右伺服慢进位置"=w720, "左伺服顶升位置"=w719, "右伺服顶升位置"=w718, "伺服慢进速度"=w717, "保压时间"=w716, "顶升压力"=w715) -> ("Result"=w714:string)  [unwired: 3 in, 1 out]
            }
            frame #1 {
              n581 = Index Array(array=w773, index #1=0 ("索引"), index #2=24 ("索引"), index #3=25 ("索引"), index #4=26 ("索引")) -> (element #1=w766:string, element #2=w770:string, element #3=w763:string, element #4=w762:string)  [unwired: 21 in, 21 out]
              n582 = call "创建文本"("产品型号"=w766, "气缸启用"=w770, "左压力换向"=w763, "右压力换向"=w762) -> ("Result"=w769:string)  [unwired: 10 in, 1 out]
              n583 = Concatenate Strings(w768, w769) -> (w767:string)
            }
          }
          n584 = call "ADO Connection Create.vi"() -> ("error out"=w708:errorcluster, "ADODB._Connection Out"=w709:refnum<k7>)  [unwired: 10 in]
          n585 = call "ADO Connection Open.vi"("error in (no error)"=w708, "ConnectionString"="DSN=参数Z120;", "ADODB._Connection In"=w709) -> ("error out"=w705:errorcluster, "ADODB._Connection Out"=w706:refnum<k7>)  [unwired: 7 in]
          n586 = call "SQL Execute.vi"("error in (no error)"=w705, "Command Text"=w701, "ADODB._Connection In"=w706) -> ("error out"=w712:errorcluster, "ADODB._Connection Out"=w713:refnum<k7>)  [unwired: 5 in, 2 out]
          n587 = call "ADO Connection Close.vi"("error in (no error)"=w712, "ADODB._Connection In"=w713) -> ("error out"=→"参数保存错误":errorcluster)  [unwired: 8 in, 1 out]
        }
      }
      event "传感器参数保存": Value Change {
        n588 = event-data() -> ()  [unwired: 1 in, 6 out]
        n589 = local read "左位移零点偏移值"() -> (w799:dbl)
        n590 = local read "左位移比例偏移值"() -> (w800:dbl)
        n591 = local read "右位移零点偏移值"() -> (w803:dbl)
        n592 = local read "右位移比例偏移值"() -> (w804:dbl)
        n593 = local read "压力1零点偏移值"() -> (w797:dbl)
        n594 = local read "压力1比例偏移值"() -> (w798:dbl)
        n595 = local read "压力2零点偏移值"() -> (w801:dbl)
        n596 = local read "压力2比例偏移值"() -> (w802:dbl)
        n597 = Number To Fractional String(number=w797, precision (6)=i16 3 ("精度(6)")) -> (F-format string=w789:string)  [unwired: 2 in]
        n598 = Number To Fractional String(number=w798, precision (6)=i16 3 ("精度(6)")) -> (F-format string=w790:string)  [unwired: 2 in]
        n599 = Number To Fractional String(number=w799, precision (6)=i16 3 ("精度(6)")) -> (F-format string=w791:string)  [unwired: 2 in]
        n600 = Number To Fractional String(number=w800, precision (6)=i16 3 ("精度(6)")) -> (F-format string=w792:string)  [unwired: 2 in]
        n601 = Number To Fractional String(number=w801, precision (6)=i16 3 ("精度(6)")) -> (F-format string=w793:string)  [unwired: 2 in]
        n602 = Number To Fractional String(number=w802, precision (6)=i16 3 ("精度(6)")) -> (F-format string=w794:string)  [unwired: 2 in]
        n603 = Number To Fractional String(number=w803, precision (6)=i16 3 ("精度(6)")) -> (F-format string=w795:string)  [unwired: 2 in]
        n604 = Number To Fractional String(number=w804, precision (6)=i16 3 ("精度(6)")) -> (F-format string=w796:string)  [unwired: 2 in]
        n605 = call "创建文本2"("左位移比例偏移值"=w792, "压力2比例偏移值"=w794, "右位移比例偏移值"=w796, "压力1零点偏移值"=w789, "压力1比例偏移值"=w790, "左位移零点偏移值"=w791, "压力2零点偏移值"=w793, "右位移零点偏移值"=w795) -> ("Result"=w805:string)  [unwired: 6 in, 1 out]
        n606 = call "ADO Connection Create.vi"() -> ("error out"=w778:errorcluster, "ADODB._Connection Out"=w776:refnum<k7>)  [unwired: 10 in]
        n607 = call "ADO Connection Open.vi"("error in (no error)"=w778, "ConnectionString"="DSN=参数Z120;", "ADODB._Connection In"=w776) -> ("error out"=w779:errorcluster, "ADODB._Connection Out"=w777:refnum<k7>)  [unwired: 7 in]
        n608 = call "SQL Execute.vi"("error in (no error)"=w779, "Command Text"=w805, "ADODB._Connection In"=w777) -> ("error out"=w775:errorcluster, "ADODB._Connection Out"=w774:refnum<k7>)  [unwired: 5 in, 2 out]
        n609 = call "ADO Connection Close.vi"("error in (no error)"=w775, "ADODB._Connection In"=w774) -> ("error out"=→"传感器保存错误":errorcluster)  [unwired: 8 in, 1 out]
      }
      event "停止": Value Change {
        n610 = event-data() -> ()  [unwired: 1 in, 6 out]
        n611 = property on="属性节点" class="App"() -> ("App.Kind"=w808:T5)  [unwired: 2 in, 2 out]
        n612 = case shown="\"Development System\"" w808 {
          tunnel: [_ w809 w810] -> w807
          frame "invalid app kind", Default {
          }
          frame "Development System" {
            w809 = TRUE ("停止？(T)")
            n613 = Stop(stop? (T)=w809) -> ()
          }
          frame "Run Time System" {
            w810 = TRUE ("退出？(T)")
            n614 = Quit LabVIEW(quit? (T)=w810) -> ()
          }
        }
      }
    }
  }
  n615 = flat-sequence {
    frame #0 {
      n616 = call "ADO Connection Create.vi"() -> ("error out"=w814:errorcluster, "ADODB._Connection Out"=w815:refnum<k7>)  [unwired: 10 in]
      n617 = call "ADO Connection Open.vi"("error in (no error)"=w814, "ConnectionString"="DSN=参数Z120;", "ADODB._Connection In"=w815) -> ("error out"=→"error out":errorcluster, "ADODB._Connection Out"=→"ADODB._Connection Out":refnum<k7>)  [unwired: 7 in]
    }
    frame #1 {
      n618 = while {
        stop <- w817 stop-if-true
        n619 = Wait Until Next ms Multiple(millisecond multiple=u32 100 ("毫秒倍数")) -> ()  [unwired: 1 out]
        n620 = First Call?() -> (First Call?: T/F=w820:bool)
        n621 = Or(x=w820, y="参数加载") -> (x .or. y?=w819:bool)
        n622 = case shown="真" w819 {
          frame False {
          }
          frame True {
            n623 = stacked-sequence {
              frame #0 {
                n624 = First Call?() -> (First Call?: T/F=w821:bool)
                n625 = case shown="真" w821 {
                  frame False {
                  }
                  frame True {
                    n626 = local read "ADODB._Connection Out"() -> (w823:refnum<k7>)
                    n627 = local read "error out"() -> (w822:errorcluster)
                    n628 = call "SQL Execute.vi"("error in (no error)"=w822, "Command Text"="SELECT * FROM 测试参数表 ;", "ADODB._Connection In"=w823) -> ("Data"=w826:string[][])  [unwired: 5 in, 3 out]
                    n629 = Index Array "索引数组"(array=w826, index (col)=0 ("禁用的索引 (列)")) -> (element=w829:string[])  [unwired: 1 in]
                    n630 = Array Size "数组大小"(array=w829) -> (size(s)=w828:i32)
                    n631 = while {
                      shift-right: [w834] -> w827
                      shift-left: i32[] [] -> [w835]
                      tunnel: w828 -> [w832]
                      i -> [w833]
                      stop <- w836 stop-if-true
                      n632 = Greater Or Equal?(x=w833, y=w832) -> (x >= y?=w836:bool)
                      n633 = Build Array (concatenate) "创建数组"(w835, w833) -> (w834:i32[])
                    }
                    n634 = Build Cluster Array "索引与捆绑簇数组"(w829, w827) -> (w824:cluster{"String":string, i32}[])
                    n635 = property on="型号选择" class="Ring (严格)"("StringsAndValues[]"=w824) -> ()  [unwired: 2 in, 2 out]
                  }
                }
              }
              frame #1 {
                n636 = property on="型号选择" class="Ring (严格)"() -> ("RingText.Text"=w841:string)  [unwired: 2 in, 2 out]
                n637 = local read "ADODB._Connection Out"() -> (w839:refnum<k7>)
                n638 = call "创建文本4"("产品型号"=w841) -> ("Result"=w843:string)  [unwired: 13 in, 1 out]
                n639 = local read "error out"() -> (w838:errorcluster)
                n640 = call "SQL Execute.vi"("error in (no error)"=w838, "Command Text"=w843, "ADODB._Connection In"=w839) -> ("error out"=w837:errorcluster, "Data"=w845:string[][])  [unwired: 5 in, 2 out]
                n641 = local write "error out"(w837) -> ()
                n642 = Index Array "索引数组"(array=w845, index (row)=0 ("索引 (行)")) -> (element=w842:string[])  [unwired: 1 in]
                n643 = Fract/Exp String To Number "分数/指数字符串至数值转换"(string=w842) -> (number=w840:dbl[])  [unwired: 3 in, 1 out]
                n644 = stacked-sequence {
                  tunnel: w840 -> [w890 w912]
                  frame #0 {
                    n645 = Index Array(array=w890, index #1=1 ("索引"), index #2=2 ("索引"), index #3=3 ("索引"), index #4=4 ("索引"), index #5=5 ("索引"), index #6=6 ("索引"), index #7=7 ("索引"), index #8=8 ("索引"), index #9=9 ("索引"), index #10=10 ("索引"), index #11=11 ("索引"), index #12=12 ("索引"), index #13=13 ("索引"), index #14=14 ("索引"), index #15=15 ("索引"), index #16=16 ("索引"), index #17=17 ("索引"), index #18=18 ("索引"), index #19=19 ("索引"), index #20=20 ("索引"), index #21=21 ("索引"), index #22=22 ("索引"), index #23=23 ("索引"), index #24=24 ("索引")) -> (element #1=w873:dbl, element #2=w872:dbl, element #3=w871:dbl, element #4=w870:dbl, element #5=w869:dbl, element #6=w868:dbl, element #7=w867:dbl, element #8=w866:dbl, element #9=w865:dbl, element #10=w864:dbl, element #11=w863:dbl, element #12=w862:dbl, element #13=w861:dbl, element #14=w860:dbl, element #15=w859:dbl, element #16=w858:dbl, element #17=w857:dbl, element #18=w856:dbl, element #19=w855:dbl, element #20=w853:dbl, element #21=w851:dbl, element #22=w876:dbl, element #23=→"顶升压力":dbl, element #24=w847:dbl)
                    n646 = To Unsigned Long Integer(number=w876) -> (unsigned 32bit integer=w850:u32)
                    n647 = local write "保压时间"(w850) -> ()
                    n648 = local write "气缸启用"(w847) -> ()
                    n649 = Multiply(x=w860, y=-1.0 ("x")) -> (x*y=w889:dbl)
                    n650 = Multiply(x=w859, y=-1.0) -> (x*y=w888:dbl)
                    n651 = Multiply(x=w857, y=-1.0) -> (x*y=w885:dbl)
                    n652 = Multiply(x=w856, y=-1.0 ("x")) -> (x*y=w883:dbl)
                    n653 = Multiply(x=w855, y=-1.0 ("x")) -> (x*y=w854:dbl)
                    n654 = Multiply(x=w853, y=-1.0 ("x")) -> (x*y=w852:dbl)
                    n655 = local write "区域最小位移(mm)"(w873) -> ()
                    n656 = local write "区域最大位移(mm)"(w872) -> ()
                    n657 = local write "区域最小压力(N)"(w871) -> ()
                    n658 = local write "区域最大压力(N)"(w870) -> ()
                    n659 = local write "监控点位移(mm)"(w869) -> ()
                    n660 = local write "左伺服压入力下限(N)"(w868) -> ()
                    n661 = local write "左伺服压入力上限(N)"(w867) -> ()
                    n662 = local write "左伺服压入深度下限(mm)"(w866) -> ()
                    n663 = local write "左伺服压入深度上限(mm)"(w865) -> ()
                    n664 = local write "右伺服压入力下限(N)"(w864) -> ()
                    n665 = local write "右伺服压入力上限(N)"(w863) -> ()
                    n666 = local write "右伺服压入深度下限(mm)"(w862) -> ()
                    n667 = local write "右伺服压入深度上限(mm)"(w861) -> ()
                    n668 = local write "左伺服快进位置"(w889) -> ()
                    n669 = local write "右伺服快进位置"(w888) -> ()
                    n670 = local write "伺服快进速度"(w858) -> ()
                    n671 = local write "左伺服慢进位置"(w885) -> ()
                    n672 = local write "右伺服慢进位置"(w883) -> ()
                    n673 = local write "左伺服顶升位置"(w854) -> ()
                    n674 = local write "右伺服顶升位置"(w852) -> ()
                    n675 = local write "伺服慢进速度"(w851) -> ()
                  }
                  frame #1 {
                    n676 = Index Array(array=w912, index #1=25 ("索引"), index #2=26 ("索引")) -> (element #1=→"左压力换向(N)":dbl, element #2=→"右压力换向(N)":dbl)  [unwired: 13 in, 13 out]
                  }
                }
              }
              frame #2 {
                n677 = local read "ADODB._Connection Out"() -> (w925:refnum<k7>)
                n678 = call "SQL Execute.vi"("Command Text"="SELECT * FROM 传感器校验表 where ID='2'", "ADODB._Connection In"=w925) -> ("Data"=w926:string[][])  [unwired: 6 in, 3 out]
                n679 = Index Array "索引数组"(array=w926) -> (element=w927:string[])  [unwired: 2 in]
                n680 = Fract/Exp String To Number "分数/指数字符串至数值转换"(string=w927) -> (number=w928:dbl[])  [unwired: 3 in, 1 out]
                n681 = Index Array "索引数组"(array=w928, index #1=1 ("索引"), index #2=2 ("索引"), index #3=3 ("索引"), index #4=4 ("索引"), index #5=5 ("索引"), index #6=6 ("索引"), index #7=7 ("索引"), index #8=8 ("索引")) -> (element #1=w920:dbl, element #2=w919:dbl, element #3=w918:dbl, element #4=w917:dbl, element #5=w916:dbl, element #6=w915:dbl, element #7=w914:dbl, element #8=w913:dbl)
                n682 = local write "左位移零点偏移值"(w918) -> ()
                n683 = local write "左位移比例偏移值"(w917) -> ()
                n684 = local write "右位移零点偏移值"(w914) -> ()
                n685 = local write "右位移比例偏移值"(w913) -> ()
                n686 = local write "压力1零点偏移值"(w920) -> ()
                n687 = local write "压力1比例偏移值"(w919) -> ()
                n688 = local write "压力2零点偏移值"(w916) -> ()
                n689 = local write "压力2比例偏移值"(w915) -> ()
              }
            }
          }
        }
        n690 = local read "停止"() -> (w817:bool)
      }
    }
    frame #2 {
      n691 = local read "ADODB._Connection Out"() -> (w934:refnum<k7>)
      n692 = call "ADO Connection Close.vi"("ADODB._Connection In"=w934) -> ("error out"=→"参数加载错误":errorcluster)  [unwired: 9 in, 1 out]
    }
  }
  n693 = flat-sequence {
    tunnel: [w936] -> w3
    tunnel: w3 -> [w938]
    tunnel: [w937] -> w2
    tunnel: w2 -> [w1006]
    tunnel: [w1006] -> w1
    tunnel: w1 -> [w1008]
    frame #0 {
      n694 = call "PCI8622配置.vi"() -> ("DeviceID"=w936:i32)  [unwired: 11 in]
    }
    frame #1 {
      n695 = while {
        tunnel: w938 -> [w967]
        tunnel: [w967] -> w937
        stop <- w958 stop-if-true
        w1004 = 0  # nRetSizeWords
        w1005 = 2048  # nReadSizeWords
        # "hDevice"
        n696 = Wait Until Next ms Multiple(millisecond multiple=u32 50 ("毫秒倍数")) -> ()  [unwired: 1 out]
        n697 = Initialize Array(u16 0, 2048 ("dimension size")) -> (w997:u16[])
        n698 = dll-call lib="PTH17abs DQ14070-Z120人机界面-Z120PCI8622_32.dll" fn="PCI8622_ReadDeviceProAD_Npt" label="ReadDeviceProAD_Npt"("hDevice"=w967, "ADBuffer[]"=w997, "nReadSizeWords"=w1005, "nRetSizeWords"=w1004) -> ("ADBuffer[]"=w1000:u16[])  [unwired: 7 in, 2 out]
        n699 = Divide(x=w1000, y=65536.01) -> (x/y=w1001:dbl[])
        n700 = Multiply(x=w1001, y=20) -> (x*y=w944:dbl[])
        n701 = Subtract(x=w944, y=10) -> (x-y=w945:dbl[])
        n702 = Decimate 1D Array "抽取一维数组"(w945) -> (w994:dbl[], w982:dbl[], w972:dbl[], w971:dbl[])
        n703 = Add Array Elements(numeric array=w972) -> (sum=w969:dbl)
        n704 = Add Array Elements(numeric array=w994) -> (sum=w940:dbl)
        n705 = Array Size(array=w972) -> (size(s)=w981:i32)
        n706 = Add Array Elements(numeric array=w982) -> (sum=w988:dbl)
        n707 = Array Size(array=w994) -> (size(s)=w995:i32)
        n708 = Array Size(array=w982) -> (size(s)=w989:i32)
        n709 = Add Array Elements(numeric array=w971) -> (sum=w968:dbl)
        n710 = Array Size(array=w971) -> (size(s)=w970:i32)
        n711 = Divide(x=w969, y=w981) -> (x/y=w980:dbl)
        n712 = Divide(x=w940, y=w995) -> (x/y=w939:dbl)
        "电压值" <- w939
        n713 = Divide(x=w988, y=w989) -> (x/y=w986:dbl)
        n714 = Divide(x=w968, y=w970) -> (x/y=w976:dbl)
        n715 = local read "压力1零点偏移值"() -> (w952:dbl)
        n716 = Subtract(x=w980, y=-0.02) -> (x-y=w962:dbl)
        n717 = local read "右位移零点偏移值"() -> (w949:dbl)
        n718 = Subtract(x=w986, y=-0.566) -> (x-y=w984:dbl)
        n719 = Subtract(x=w976, y=0.0) -> (x-y=w960:dbl)
        n720 = Subtract(x=w939, y="压力零点标定") -> (x-y=w991:dbl)
        n721 = local read "压力2零点偏移值"() -> (w955:dbl)
        n722 = local read "左位移零点偏移值"() -> (w951:dbl)
        n723 = Multiply(x=w984, y=1000.0) -> (x*y=w983:dbl)
        n724 = Multiply(x=w991, y=2000.0) -> (x*y=w990:dbl)
        n725 = Subtract(x=w983, y=w952) -> (x-y=w946:dbl)
        n726 = Multiply(x=w960, y=25.0) -> (x*y=w973:dbl)
        n727 = Multiply(x=w962, y=25.0) -> (x*y=w977:dbl)
        n728 = local read "压力1比例偏移值"() -> (w953:dbl)
        n729 = Subtract(x=w990, y=w955) -> (x-y=w947:dbl)
        n730 = local read "右位移比例偏移值"() -> (w948:dbl)
        n731 = Subtract(x=w973, y=w951) -> (x-y=w959:dbl)
        n732 = Subtract(x=w977, y=w949) -> (x-y=w961:dbl)
        n733 = local read "压力2比例偏移值"() -> (w954:dbl)
        n734 = local read "左位移比例偏移值"() -> (w950:dbl)
        n735 = Multiply(x=w946, y=w953) -> (x*y=w942:dbl)
        n736 = Multiply(x=w961, y=w948) -> (x*y=w957:dbl)
        n737 = Multiply(x=w947, y=w954) -> (x*y=w941:dbl)
        n738 = Multiply(x=w959, y=w950) -> (x*y=w956:dbl)
        n739 = Greater Or Equal?(x=w942, y=30000.0) -> (x >= y?=→"压力报警2":bool)
        n740 = local write "右实时位移(mm)"(w957) -> ()
        n741 = local write "右实时压力(N)"(w942) -> ()
        n742 = local write "左实时压力(N)"(w941) -> ()
        n743 = local write "左实时位移(mm)"(w956) -> ()
        n744 = Greater Or Equal?(x=w941, y=30000.0) -> (x >= y?=→"压力报警1":bool)
        n745 = local read "停止"() -> (w958:bool)
      }
    }
    frame #2 {
      n746 = dll-call lib="PTH17abs DQ14070-Z120人机界面-Z120PCI8622_32.dll" fn="PCI8622_StopDeviceProAD" label="StopDeviceProAD"("hDevice"=w1006) -> ("hDevice"=w1007:i32)  [unwired: 4 in, 2 out]
      n747 = dll-call lib="PTH17abs DQ14070-Z120人机界面-Z120PCI8622_32.dll" fn="PCI8622_ReleaseDeviceProAD" label="ReleaseDeviceProAD"("hDevice"=w1007) -> ()  [unwired: 5 in, 2 out]
    }
    frame #3 {
      n748 = dll-call lib="PTH17abs DQ14070-Z120人机界面-Z120PCI8622_32.dll" fn="PCI8622_ReleaseDevice" label="ReleaseDevice"("hDevice"=w1008) -> ()  [unwired: 5 in, 2 out]
    }
  }
